vi "Custom Device CORE.vi"(8 "error in (no error)":errorcluster, 11 "CDW_MetaDataObj":refnum<class "NIVS_Consolidated_CDW_MetaDataObj.lvclass">) -> (0 "error out":errorcluster)   [LabVIEW 2020, in "NIVS_Consolidated_CDW_MetaDataObj.lvclass"]
doc: "This VI is the Core VI for the Custom Device Wizard.\n\nWritten by:\nStephan Daunke\n\nDate:\n2014/01/27\n\nCompany:\nNational Instruments Germany GmbH"
uses:
  NIVS_Consolidated_CDW_MetaDataObj.lvclass
  C:/Program Files/National Instruments/LabVIEW 2024/resource/dialog/NewProjectWizard/MetaDataObj/MetaDataObj.lvclass
  Action.ctl
  Internal data.ctl
  <resource>/dialog/NewProjectWizard/MetaDataObj/MetaDataObj.lvclass/MetaDataObj.ctl
  NIVS_Consolidated_CDW_MetaDataObj.lvclass/NIVS_Consolidated_CDW_MetaDataObj.ctl
  Template Classes/NIVS_CD Template/NIVS_CD Template.lvclass/NIVS_CD Template.ctl
  Template Classes/NIVS_PPLCD Template/NIVS_PPLCD Template.lvclass
  Utility folder.ctl
  CD Shared lvlib.ctl
  Common.ctl
  Add Item - Type.ctl
  CD System Explorer lvlib.ctl
  <vilib>/Utility/traverseref.llb/TRef TravTarget.ctl
  CD Engine lvlib.ctl
  Build Spec System Explorer.ctl
  Build Spec Engine.ctl
  <resource>/dialog/NewProjectWizard/MetaDataObj/Accessors/Read Project Root.vi
  Read CD Template.vi
  Template Classes/NIVS_CD Template/Read Extra Page Names.vi
  <resource>/dialog/NewProjectWizard/MetaDataObj/Accessors/Read Project Name.vi
  Template Classes/NIVS_CD Template/Read Support Runtime Configuration.vi
  Utility folder.vi
  CD Shared lvlib.vi
  Common.vi
  CD System Explorer lvlib.vi
  CD Engine lvlib.vi
  Build Spec System Explorer.vi
  Build Spec Engine.vi
  Template Classes/NIVS_CD Template/NIVS_CD Template.lvclass
  <vilib>/Utility/Data Type/NI_Data Type.lvlib
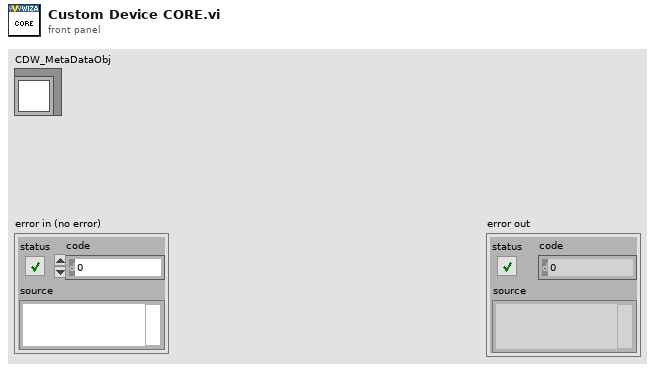
[diagram p1: front panel]
types:
  T1 = typedef "NIVS_Consolidated_CDW_MetaDataObj.lvclass/Internal data.ctl" = cluster{"CD GUID":string, "Extra Page GUIDs":string[], "System Explorer Library":refnum<vi>, "Shared Library":refnum<vi>, "Engine Library":refnum<vi>}
  T2 = typedef "NIVS_Consolidated_CDW_MetaDataObj.lvclass/Action.ctl" = enum16{"Project - Create Custom Device folder", "PC - Create GUID for each extra page", "PC-Utility - Create folder and copy -Copy .LLB to NI VeriStand dir-", "PC-Utility - Change -Copy .LLB to NI VeriStand dir-", "PC-Shared - Create folder and copy Constants.vi", "PC-Shared - Change Constants.vi content", "PC-Shared - Create library", "PC-Shared - Add folders and VIs to library", "PC-System Explorer - Create folder and copy templates", "PC-System Explorer - Create extra pages", "PC-System Explorer - Create library", "PC-System Explorer - Add folders and VIs to library", "PC-Engine - Create folder and copy the RT Template", "PC-Engine - Create library", "PC-Engine - Add virtual folders and VIs to library", "PC-XML - Create and change file", "PC-Help - Copy HTML Files", "Project - Read project file content", "Project - Edit Utility section", "Project - Edit XML section", "Project - Edit Engine Library section", "Project - Edit Shared Library section", "Project - Edit System Explorer Library section", "Project - Edit Custom Device Name", "Project - Edit System Explorer LLB Name", "Project - Edit Engine LLB OS dependent file name", "Project - Copy Configuration file", "Project - Write new project file"}
  T3 = typedef "NIVS_Consolidated_CDW_MetaDataObj.lvclass/Utility folder.ctl" = enum16{"Utility.FolderName", "Utility.PPL Tools Folder Path", "Utility.Copy .llb to NI VeriStand dir.FileName", "Utility.Copy .llb to NI VeriStand dir.FilePathAndName", "Utility.LLB Pre Build.FilePathAndName", "Utility.PPL Pre Build.FileName", "Utility.XMLUpdater.FileName", "Utility.XMLUpdater.FolderName", "Utility.XMLUpdater.Library.FileName"}
  T4 = typedef "NIVS_Consolidated_CDW_MetaDataObj.lvclass/CD Shared lvlib.ctl" = enum16{"LibraryFileName", "LibraryFolderName", "ConstantsVI.VIPathAndName", "Shared.FolderName", "Shared.Types.FolderName", "Shared.Constants.VIName", "Shared.Constants.VITemplateName", "Shared.Constants.VITemplatePathAndName", "Shared.CompiledSettings.RelativePath", "Shared.Constants.RelativePath", "Shared.CompiledSettings.Name", "Shared.CompiledSettings.Name.NoExtension", "Shared.CompiledSettings.ClusterName"}
  T5 = typedef "NIVS_Consolidated_CDW_MetaDataObj.lvclass/Common.ctl" = enum16{"ProjectName", "TemplatesFolderName", "PPLTemplatesFolderName", "ProjectTemplatePathAndName", "ProjectPPLTemplatePathAndName", "TimingAndSyncFolderName", "CustomDeviceFolderName", "PathToTemplates", "PathToPPLTemplates", "PathToExplorerPPLTemplates", "PathToEnginePPLTemplates", "PathToConfigurationFile", "ProjectConfigurationName"}
  T6 = typedef "NIVS_Consolidated_CDW_MetaDataObj.lvclass/Add Item - Type.ctl" = string
  T7 = typedef "NIVS_Consolidated_CDW_MetaDataObj.lvclass/CD System Explorer lvlib.ctl" = enum16{"LibraryFileName", "LibraryFolderName", "System Explorer.FolderName", "System Explorer.Dynamically Called.FolderName", "System Explorer.Dynamically Called.Extra Pages.FolderName", "System Explorer.Dynamically Called.Extra Pages.TemplatePathAndName", "System Explorer.Dynamically Called.Main Page.VIName", "System Explorer.Dynamically Called.Main Page.TemplatePathAndName", "System Explorer.Dynamically Called.Initialization VI.VIName", "System Explorer.Dynamically Called.Initialization VI.TemplatePathAndName", "System Explorer.SubVI.FolderName", "System Explorer.Types.FolderName", "System Explorer.ActionVIOnCompile.VIName", "System Explorer.ActionVIOnRecompile.VIName", "System Explorer.ExportConfigRTM.VIName", "System Explorer.PPL.ExportConfigRTM.VIName", "System Explorer.LoadHelpFile.VIName", "System Explorer.PPL.LoadHelpFile.VIName", "System Explorer.SetRTDriverVIsFilePaths.VIName", "System Explorer.ClearRTDriverVIs.VIName"}
  T8 = typedef "TRef TravTarget.ctl" = enum16{"FP", "BD", "Other"}
  T9 = typedef "NIVS_Consolidated_CDW_MetaDataObj.lvclass/CD Engine lvlib.ctl" = enum16{"LibraryFileName", "LibraryFolderName", "Engine.FolderName", "Engine.Init.FolderName", "Engine.Run.FolderName", "Engine.Shutdown.FolderName", "Types.FolderName", "Engine.RT Driver VI.TemplatePath", "Engine.RT Driver VI.FileName", "Engine.PPL.RT Driver VI_InlineAsync.FileName", "Engine.RTStateVariables.Name", "Engine.PPL.RTStateVariables.Name", "Engine.RTStateVariables.Name.NoExtension", "Engine.Async.NameExtension", "Engine.Async.TemplateName", "Engine.PPL.Async.TemplateName", "Engine.PPL.Async.InitVSGlobals.Name", "Engine.PPL.RT Driver VI_Inline.FileName"}
  T10 = typedef "NIVS_Consolidated_CDW_MetaDataObj.lvclass/Build Spec System Explorer.ctl" = enum16{"Destinations.LLBFileName", "Destinations.PPLFileName"}
  T11 = typedef "NIVS_Consolidated_CDW_MetaDataObj.lvclass/Build Spec Engine.ctl" = enum16{"Destinations.LLBWindowsFileName", "Destinations.LLBLinux64FileName", "Destinations.PPLWindowsFileName", "Destinations.PPLLinux64FileName"}
  T12 = enum16{"open", "replace", "create", "open or create", "replace or create", "replace or create with confirmation"}
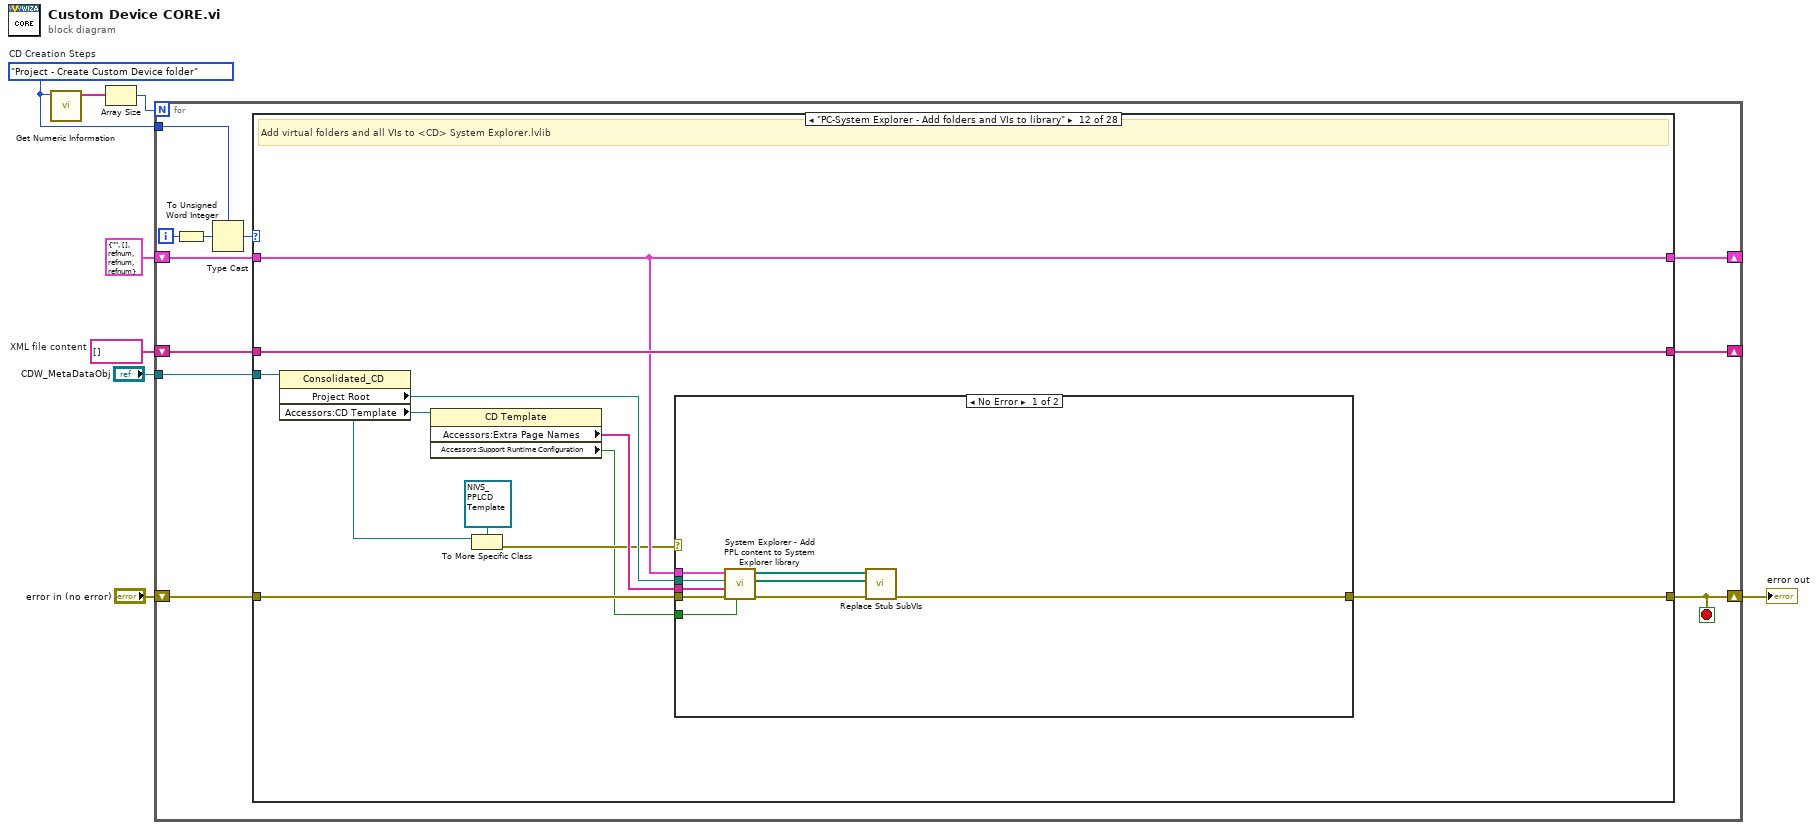
[diagram p0: block diagram]
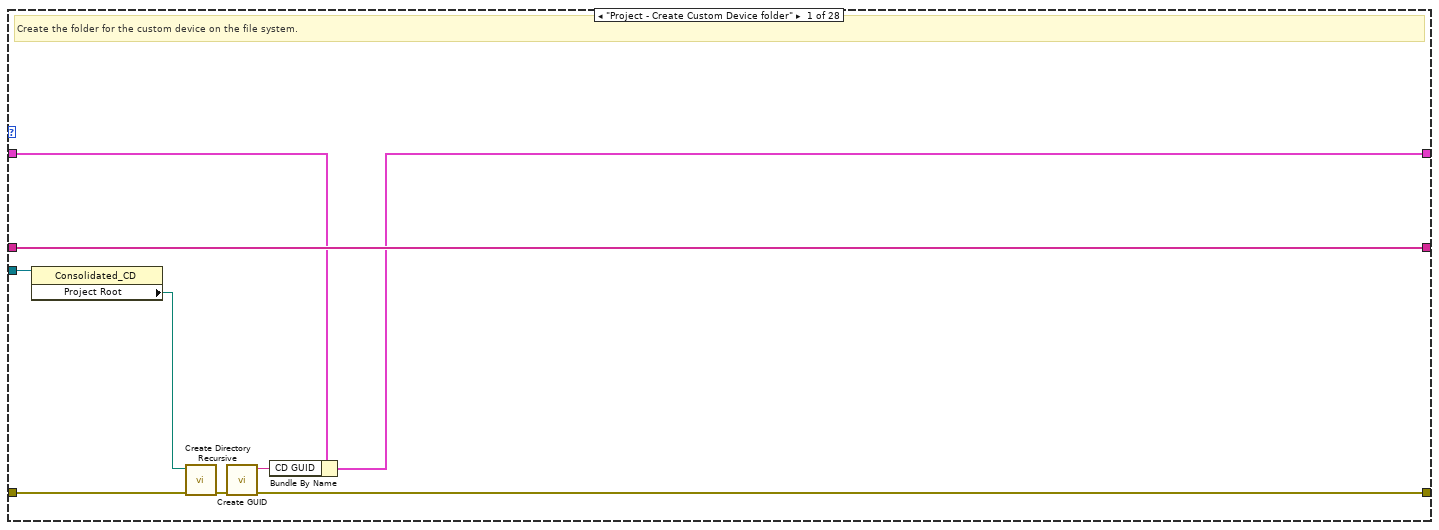
[diagram p2: hidden frame]
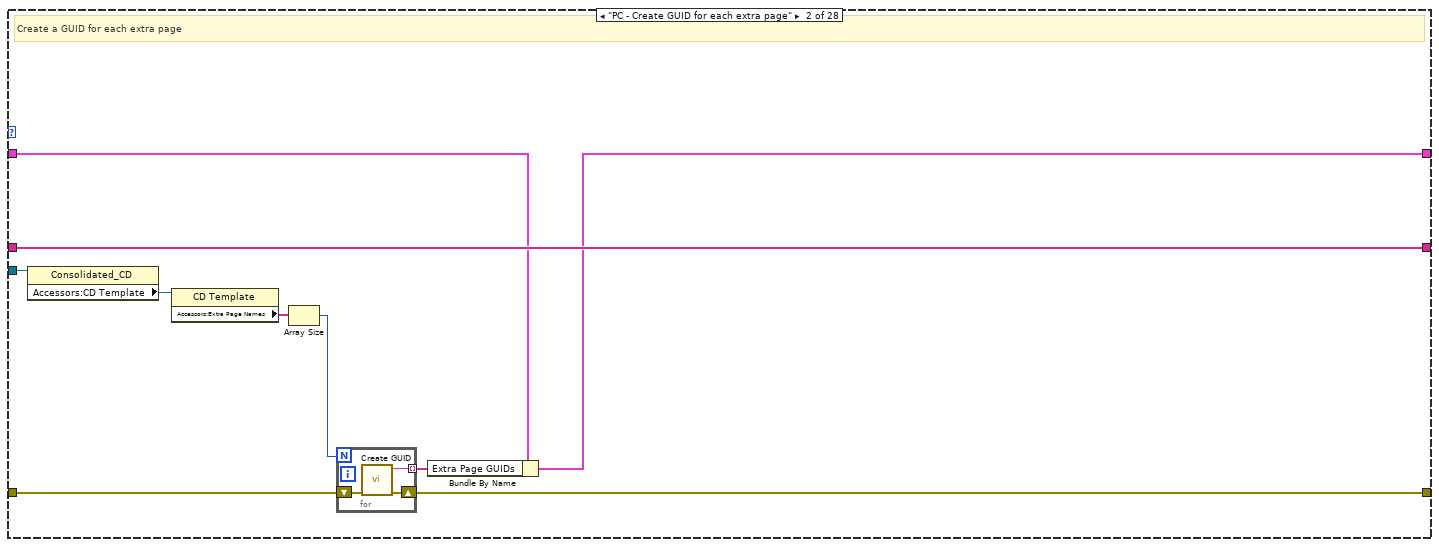
[diagram p3: hidden frame]
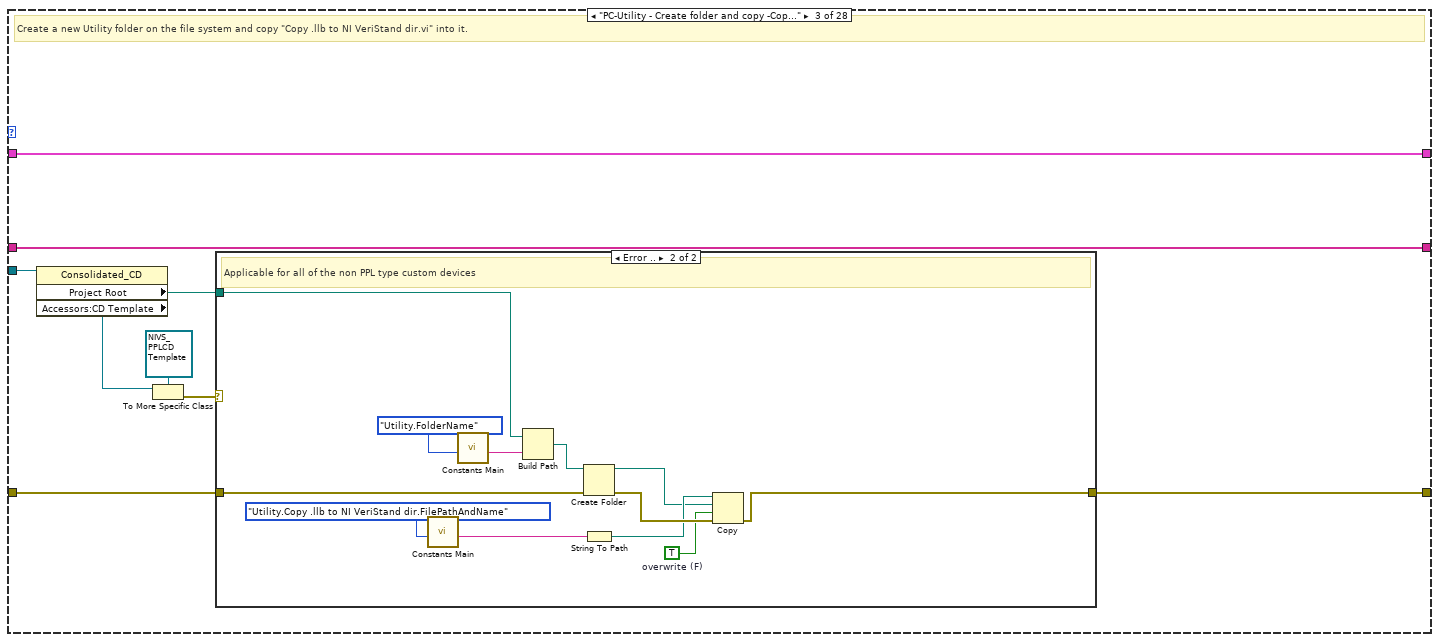
[diagram p4: hidden frame]
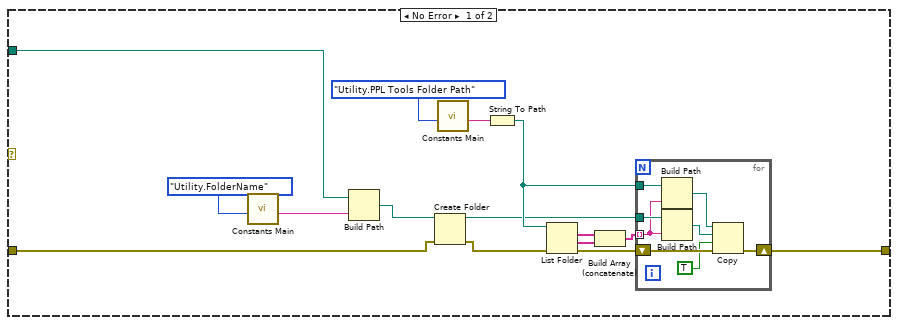
[diagram p5: hidden frame]
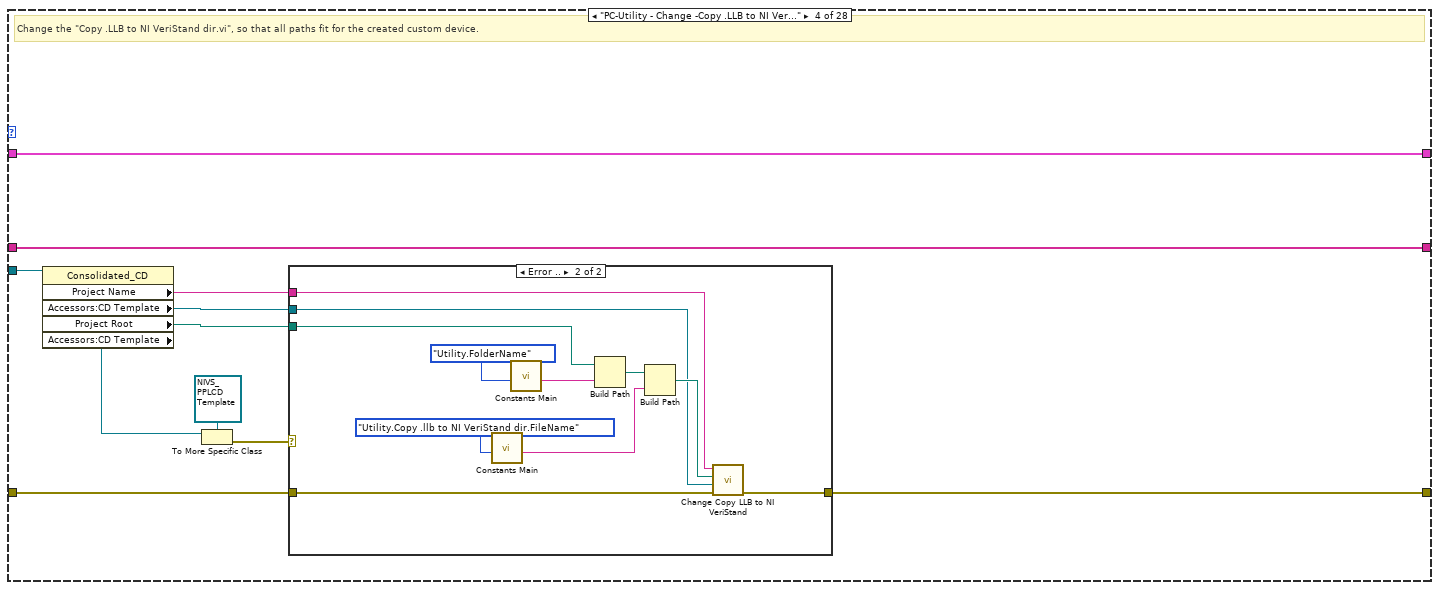
[diagram p6: hidden frame]
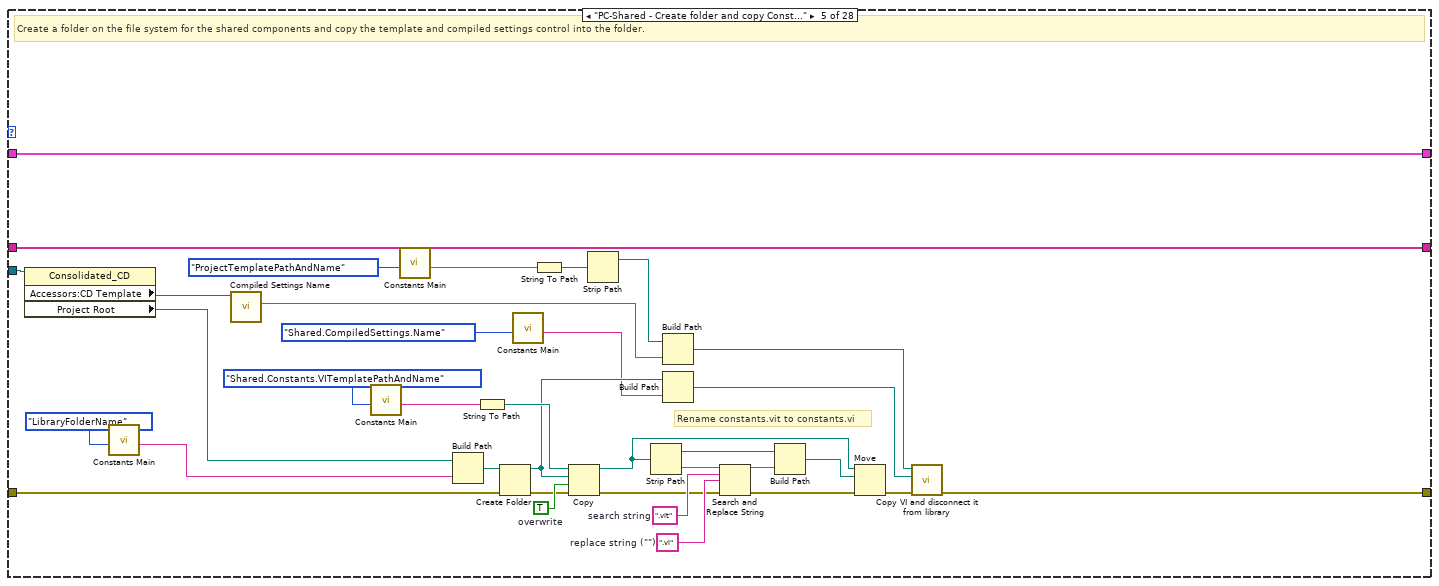
[diagram p8: hidden frame]
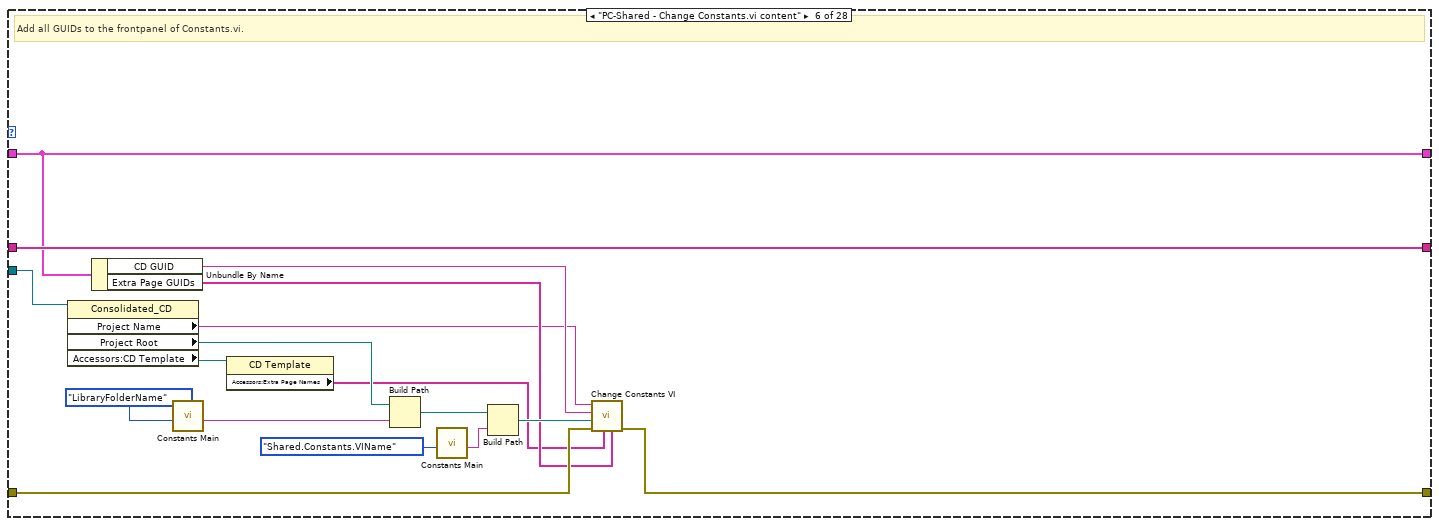
[diagram p9: hidden frame]
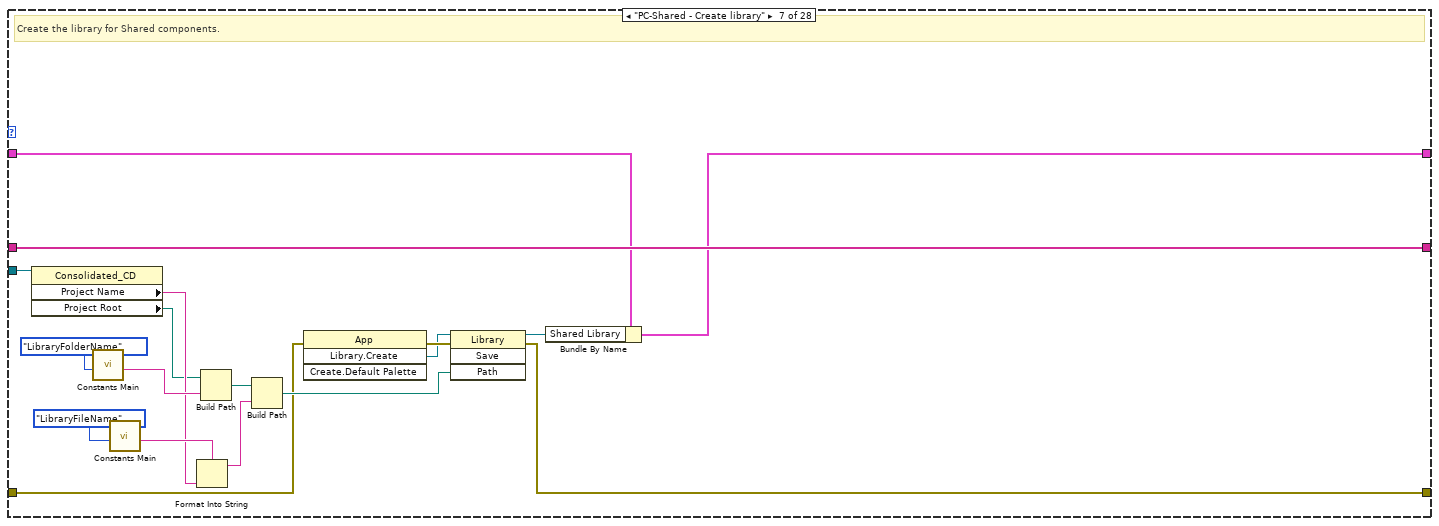
[diagram p10: hidden frame]
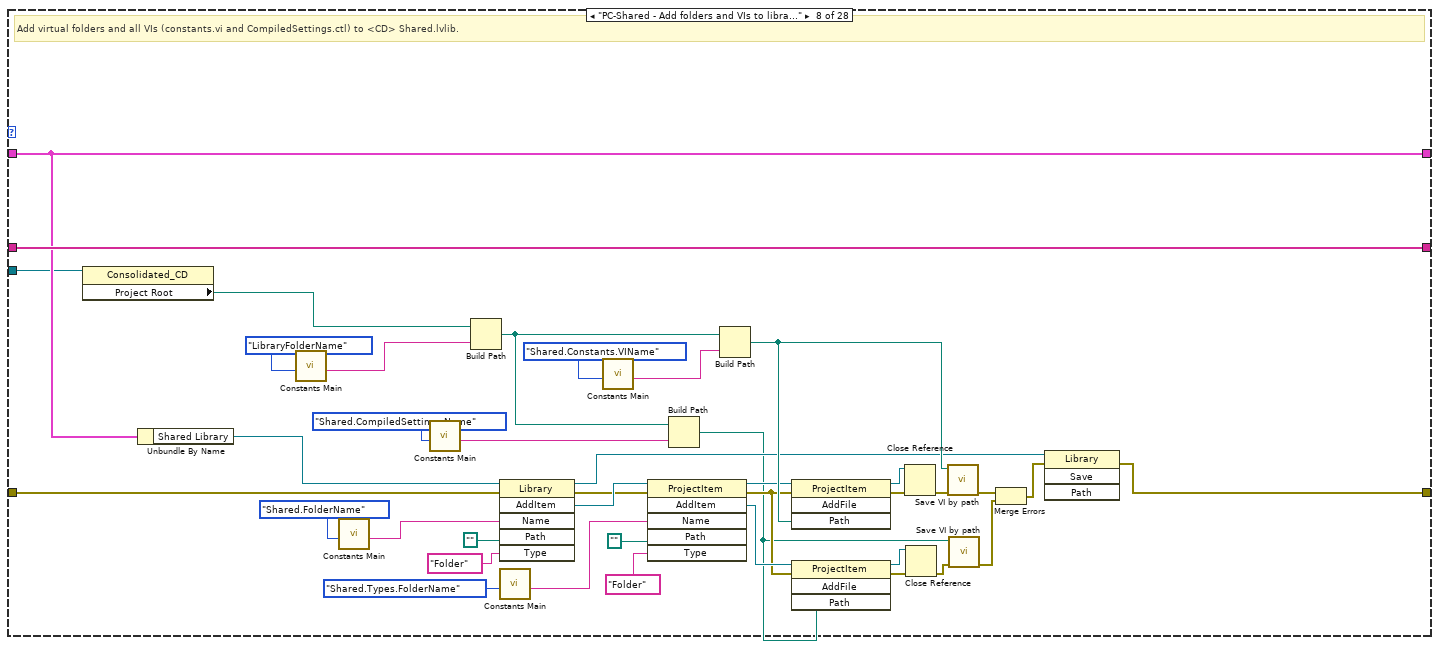
[diagram p11: hidden frame]
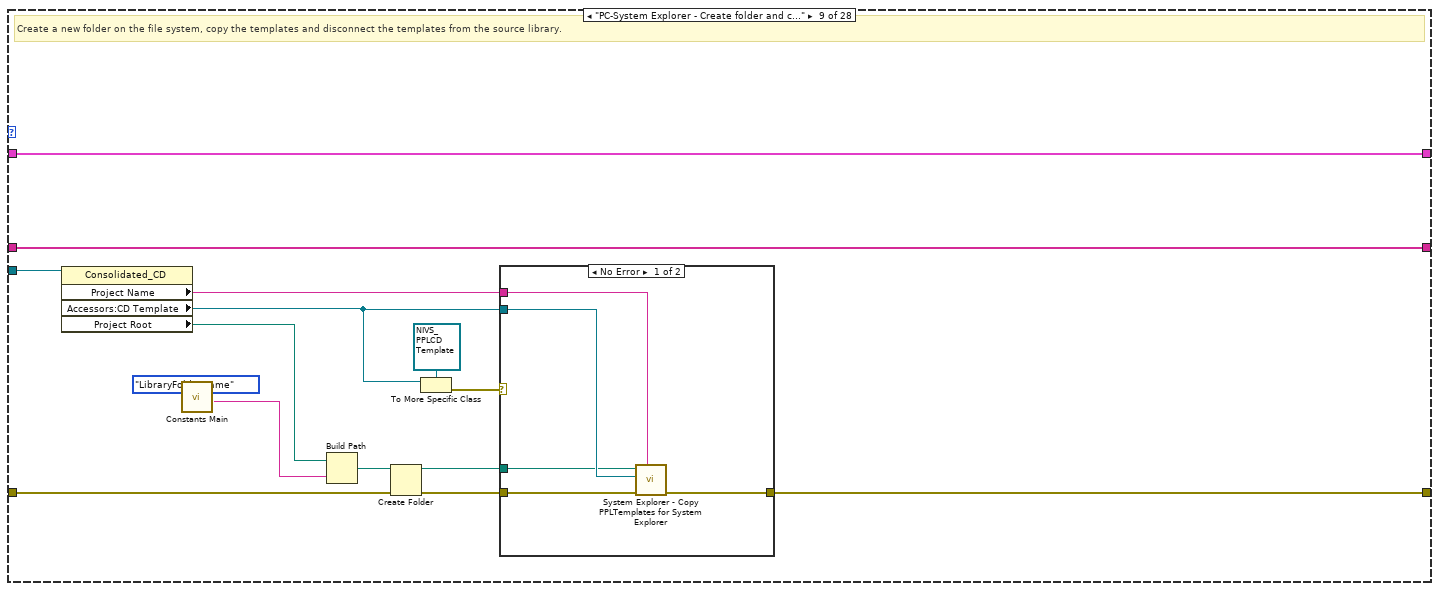
[diagram p12: hidden frame]
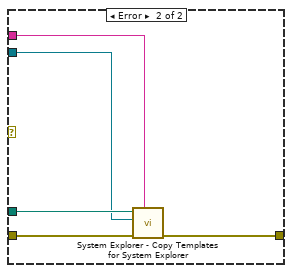
[diagram p13: hidden frame]
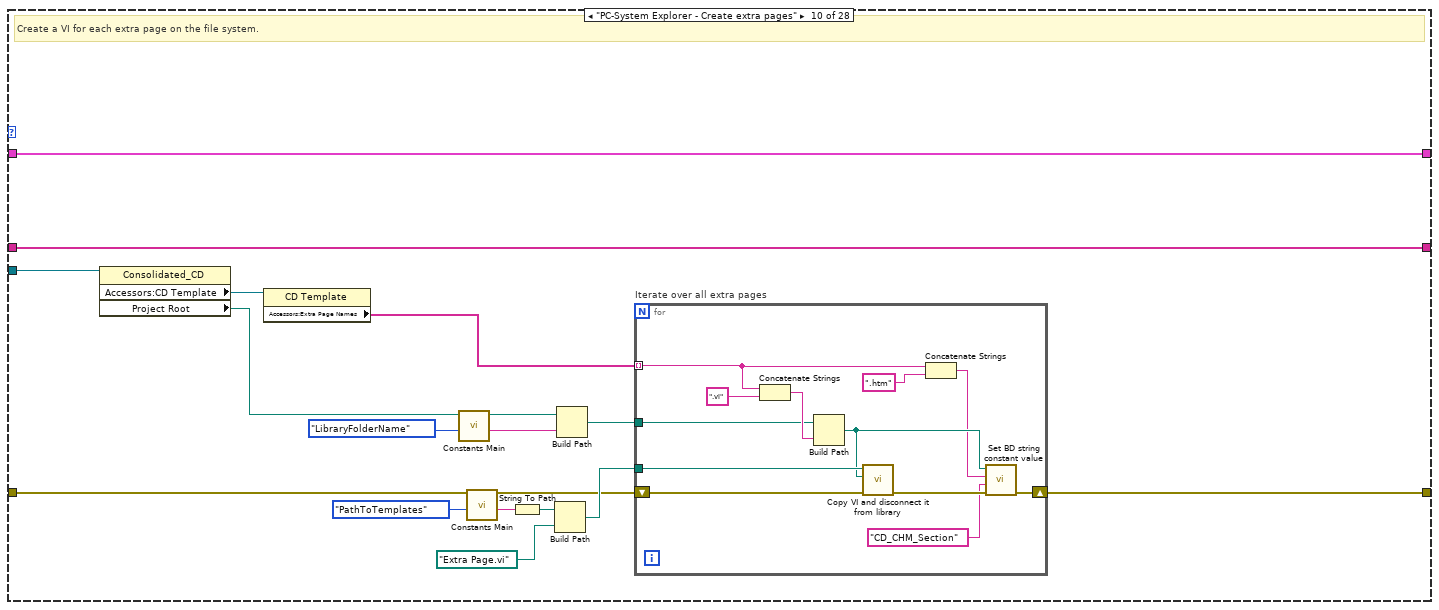
[diagram p14: hidden frame]
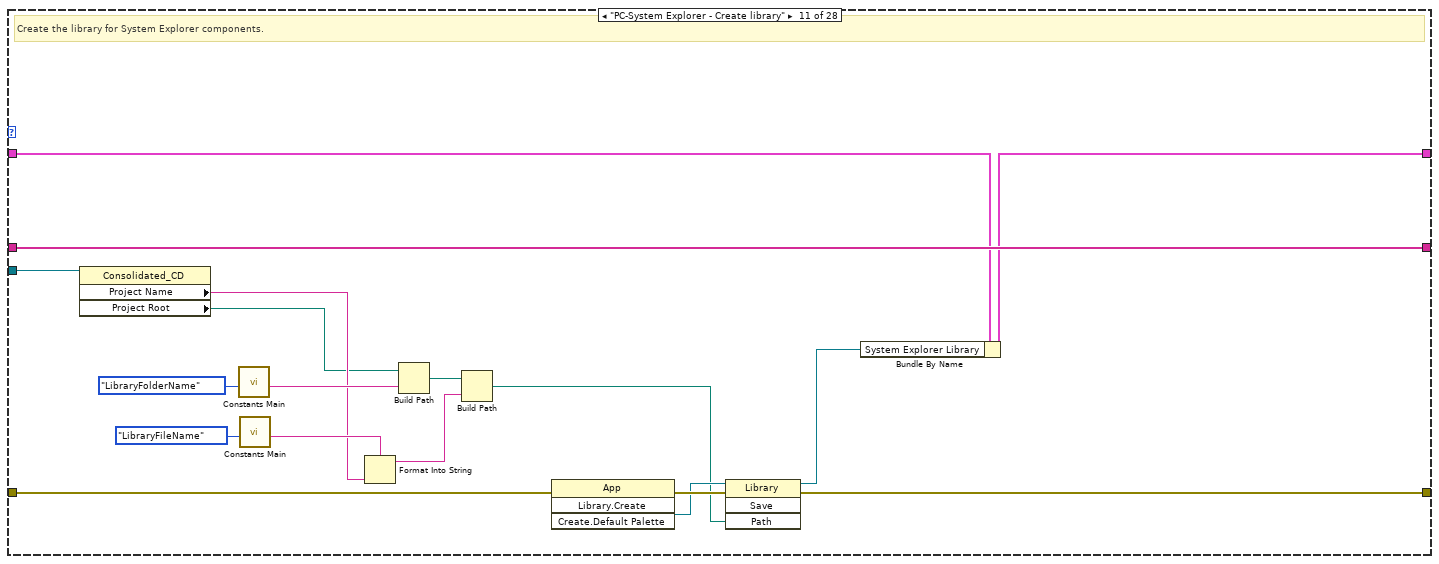
[diagram p15: hidden frame]
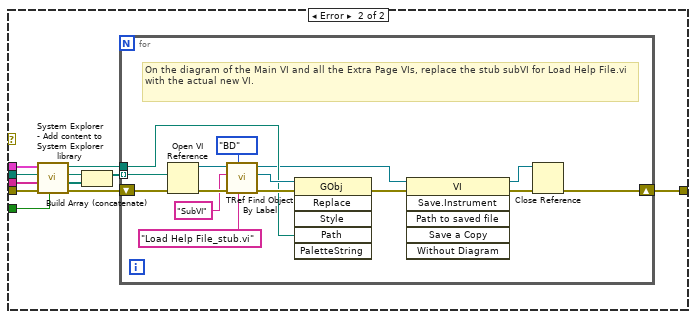
[diagram p16: hidden frame]
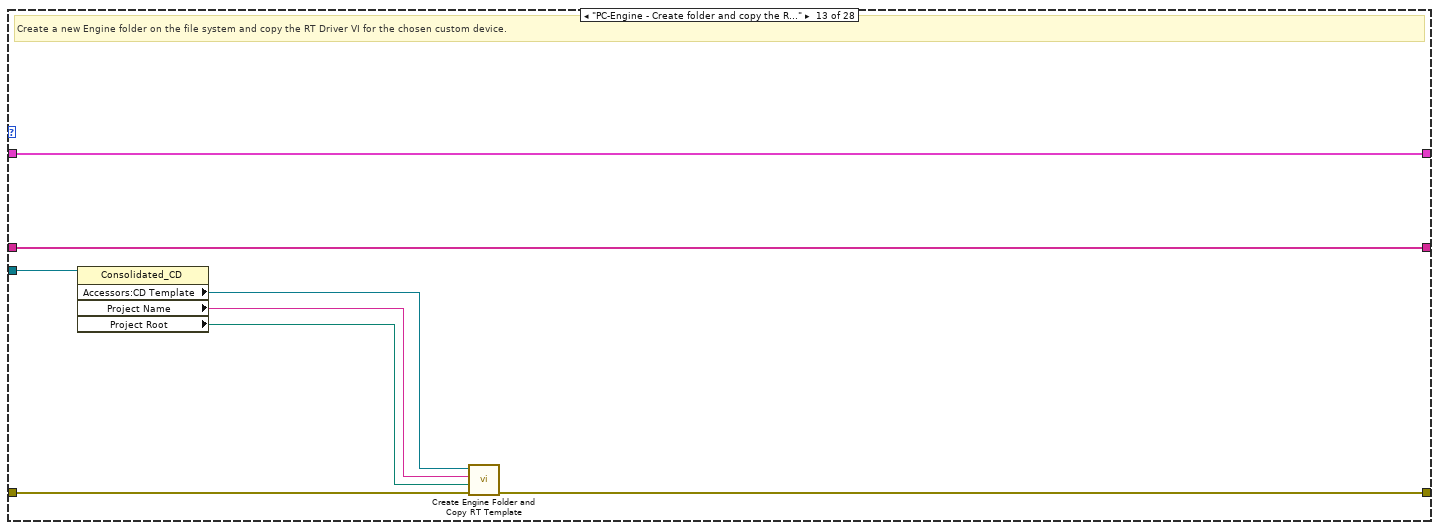
[diagram p17: hidden frame]
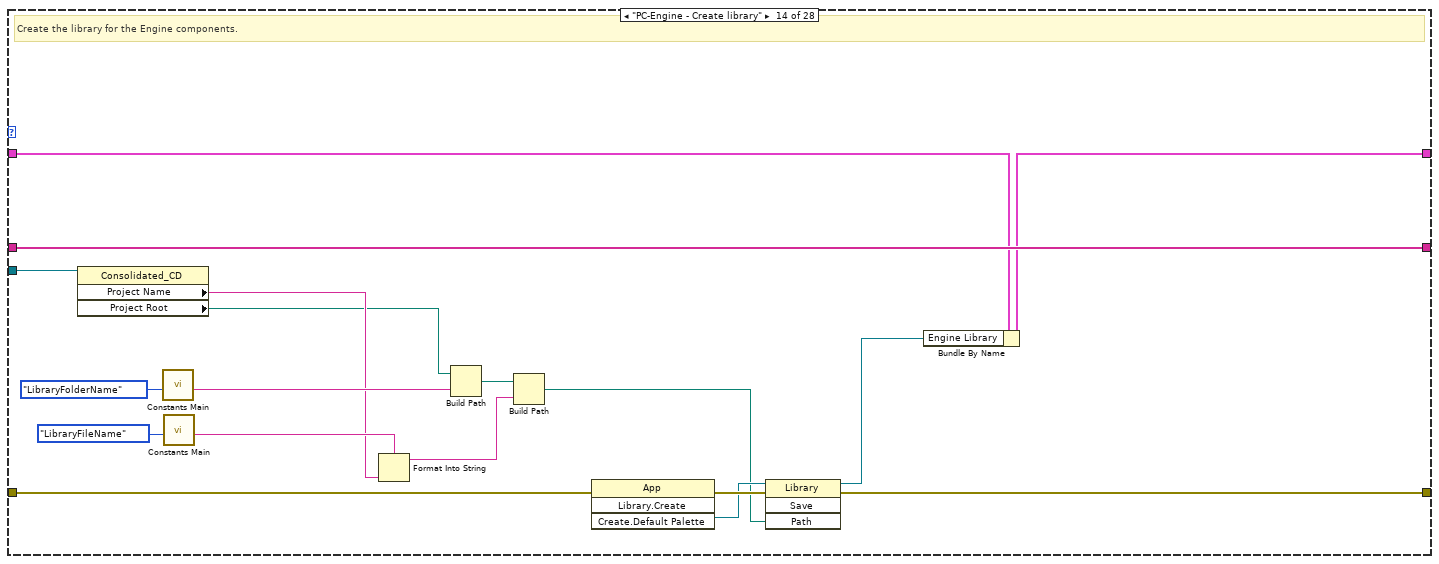
[diagram p18: hidden frame]
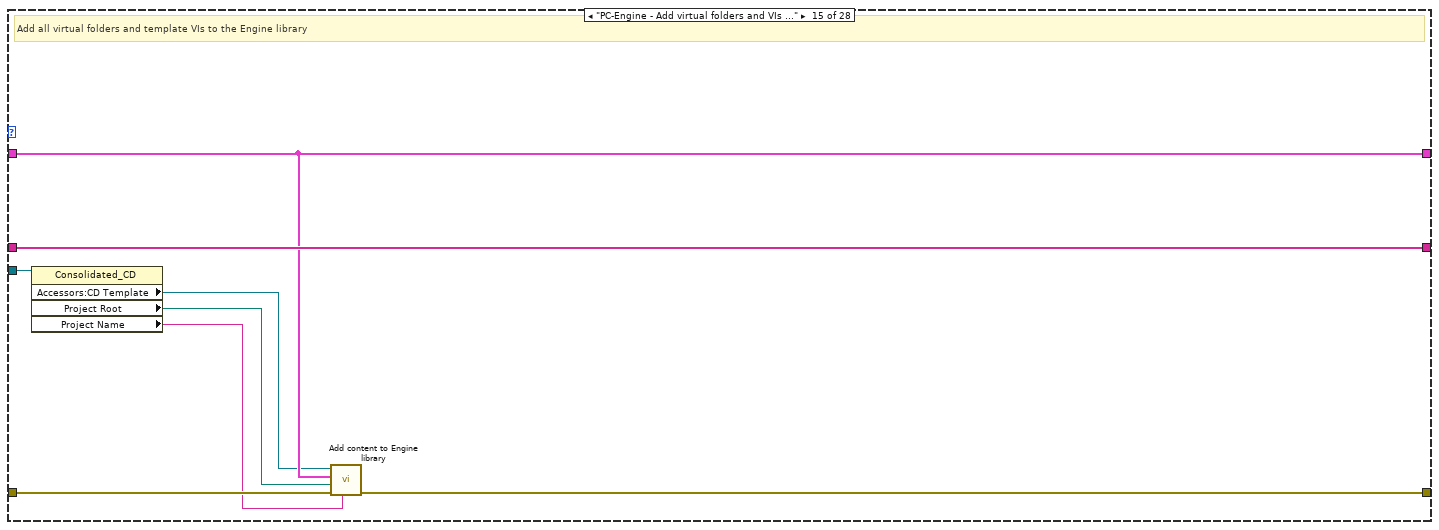
[diagram p19: hidden frame]
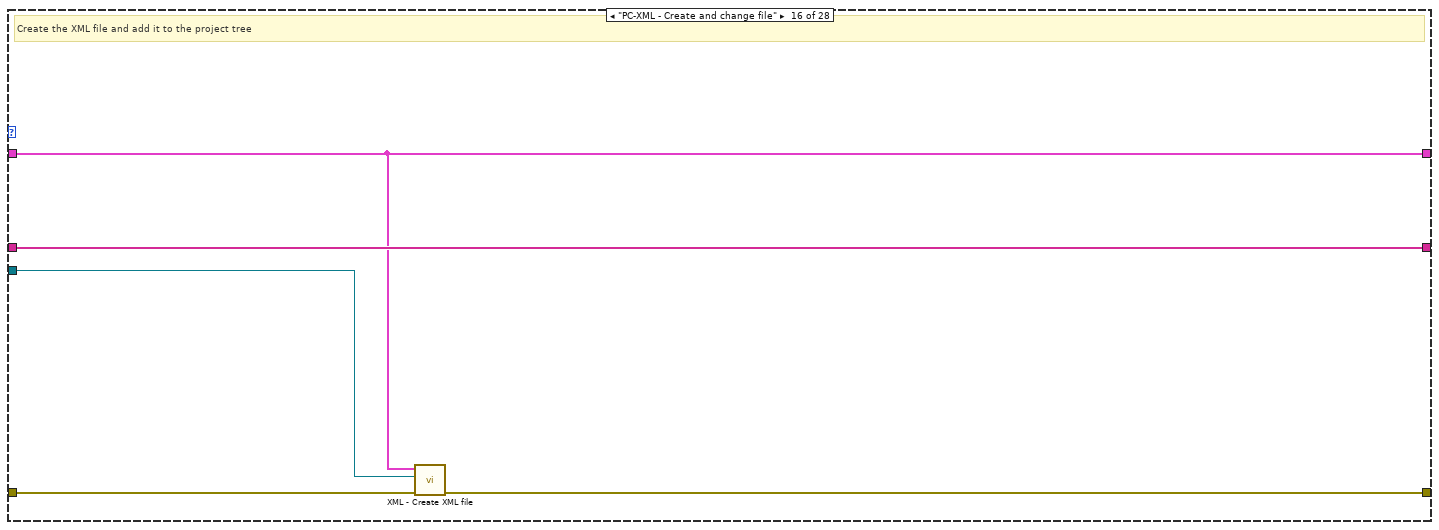
[diagram p20: hidden frame]
diagram:
  w4 = Action."Project - Create Custom Device folder"  # CD Creation Steps
  w5 = string[] []  # XML file content
  n1 = call <vilib>:"Get Numeric Information.vi"("variant"=w4) -> ("enum names"=w3:string[])  [unwired: 7 in, 3 out]
  n2 = Array Size(array=w3) -> (size(s)=w2:i32)
  n3 = for {
    N: w2 -> [_]
    shift-right: [w16] -> _
    shift-left: T1 {"CD GUID"="", "Extra Page GUIDs"=[], "System Explorer Library"=refnum, "Shared Library"=refnum, "Engine Library"=refnum} ("CD Wizard - Internal Data") -> [w18]
    shift-right: [w15] -> _
    shift-left: w5 -> [w17]
    shift-right: [w14] -> w6
    shift-left: "error in (no error)" -> [w19]
    tunnel: w4 -> [w12]
    tunnel: "CDW_MetaDataObj" -> [w11]
    i -> [w13]
    stop <- w14 stop-if-true
    n4 = To Unsigned Word Integer(number=w13) -> (unsigned 16bit integer=w10:u16)
    n5 = Type Cast(type=w12, x=w10) -> (*(type *) &x=w9:T2)
    n6 = case shown="\"PC-System Explorer - Add folders and VIs to library\"" w9 {
      tunnel: w19 -> [w24 w37 w46 w91 w113 w153 w164 w181 w223 w247 w274 w298 w341 w346 w367 w372 w387 w406 w428 w485 w504 w508 w539 w572 w586 w629 w687 w705]
      tunnel: [w25 w36 w49 w95 w115 w159 w165 w179 w218 w257 w275 w290 w335 w349 w361 w369 w378 w400 w421 w490 w503 w518 w542 w571 w590 w630 w686 w712] -> w14
      tunnel: w18 -> [w22 w34 w48 w94 w114 w150 w168 w199 w226 w256 w280 w297 w340 w353 w365 w371 w383 w416 w429 w487 w502 w509 w540 w568 w589 w632 w699 w736]
      tunnel: w17 -> [w28 w38 w50 w96 w143 w160 w178 w217 w232 w258 w288 w299 w342 w360 w368 w373 w392 _ w424 w489 w501 w513 w541 w569 w588 w631 w698 w730]
      tunnel: [w27 w33 w48 w94 w114 w150 w167 w199 w226 w256 w281 w297 w340 w352 w365 w371 w383 w416 w429 w487 w502 w509 w540 w568 w589 w632 w699 w736] -> w16
      tunnel: [w28 w38 w50 w96 w143 w160 w178 w217 w232 w258 w288 w299 w342 w360 w368 w373 w392 w410 w422 w488 w505 w519 w536 w570 w587 w627 w698 w730] -> w15
      tunnel: w11 -> [w21 w32 w45 w93 w112 w152 w163 w183 w225 w246 w273 w296 w339 w345 w366 w370 w377 w405 w425 w484 w500 w507 w538 w567 w583 w625 w692 w704]
      frame "Project - Create Custom Device folder" {
        # "Create the folder for the custom device on the file system."
        n7 = property class="Consolidated_CD"(reference=w21) -> ("Project Root"=w20:path)  [unwired: 1 in, 2 out]
        n8 = call <vilib>:"Create Directory Recursive.vi"("error in (no error)"=w24, "directory"=w20) -> ("error out"=w23:errorcluster)  [unwired: 3 in, 2 out]
        n9 = call "Create GUID.vi"("error in (no error)"=w23) -> ("error out"=w25:errorcluster, "Generated GUID"=w26:string)  [unwired: 9 in]
        n10 = Bundle By Name(cluster=w22, "CD GUID"=w26) -> (w27:T1)
      }
      frame "PC - Create GUID for each extra page" {
        # "Create a GUID for each extra page"
        n11 = property class="Consolidated_CD"(reference=w32) -> ("Accessors:CD Template"=w31:refnum<class "NIVS_CD Template.lvclass">)  [unwired: 1 in, 2 out]
        n12 = property class="CD Template"(reference=w31) -> ("Accessors:Extra Page Names"=w30:string[])  [unwired: 1 in, 2 out]
        n13 = Array Size(array=w30) -> (size(s)=w29:i32)
        n14 = for {
          N: w29 -> [_]
          shift-right: [w40] -> w36
          shift-left: w37 -> [w41]
          tunnel: [w39] -> w35 mode=indexing
          n15 = call "Create GUID.vi"("error in (no error)"=w41) -> ("error out"=w40:errorcluster, "Generated GUID"=w39:string)  [unwired: 9 in]
        }
        n16 = Bundle By Name(cluster=w34, "Extra Page GUIDs"=w35) -> (w33:T1)
      }
      frame "PC-Utility - Create folder and copy -Copy .LLB to NI VeriStand dir-" {
        # "Create a new Utility folder on the file system and copy \"Copy .llb to NI VeriStand dir.vi\" into it."
        n17 = property class="Consolidated_CD"(reference=w45) -> ("Project Root"=w47:path, "Accessors:CD Template"=w42:refnum<class "NIVS_CD Template.lvclass">)  [unwired: 1 in, 2 out]
        n18 = To More Specific Class(target class=refnum<class "NIVS_PPLCD Template.lvclass"> refnum ("NIVS_PPLCD Template.lvclass"), reference=w42) -> (error out=w43:errorcluster)  [unwired: 1 in, 1 out]
        n19 = case shown="Error .." w43 {
          tunnel: [w51 w74] -> w49
          tunnel: w47 -> [w59 w76]
          tunnel: w46 -> [w60 w75]
          frame No Error {
            n20 = call-poly "Constants Main.vi"("Action"=Utility_folder."Utility.FolderName") -> ("Output"=w61:string)  [unwired: 10 in]
            n21 = Build Path(base path=w59, name or relative path=w61) -> (appended path=w65:path)
            n22 = Create Folder(path (use dialog)=w65, error in=w60) -> (created path=w56:path, error out=w55:errorcluster)  [unwired: 1 in, 1 out]
            n23 = call-poly "Constants Main.vi"("Action"=Utility_folder."Utility.PPL Tools Folder Path") -> ("Output"=w63:string)  [unwired: 10 in]
            n24 = String To Path(string=w63) -> (path=w57:path)
            n25 = List Folder(path=w57, error in=w55) -> (filenames=w54:string[], folder names=w53:string[], error out=w58:errorcluster)  [unwired: 2 in, 1 out]
            n26 = Build Array (concatenate)(w54, w53) -> (w52:string[])
            n27 = for {
              tunnel: w52 -> [w68] mode=indexing
              tunnel: w57 -> [w71]
              shift-right: [w72] -> w51
              shift-left: w58 -> [w73]
              tunnel: w56 -> [w69]
              n28 = Build Path(base path=w71, name or relative path=w68) -> (appended path=w70:path)
              n29 = Build Path(base path=w69, name or relative path=w68) -> (appended path=w67:path)
              n30 = Copy(8:w73, 9:TRUE ("overwrite (F)"), 10:w67, 11:w70) -> (0:w72:errorcluster)  [unwired: 1 in, 2 out]
            }
          }
          frame Error {
            w83 = TRUE  # overwrite (F)
            # "Applicable for all of the non PPL type custom devices"
            n31 = call-poly "Constants Main.vi"("Action"=Utility_folder."Utility.Copy .llb to NI VeriStand dir.FilePathAndName") -> ("Output"=w81:string)  [unwired: 10 in]
            n32 = call-poly "Constants Main.vi"("Action"=Utility_folder."Utility.FolderName") -> ("Output"=w78:string)  [unwired: 10 in]
            n33 = Build Path(base path=w76, name or relative path=w78) -> (appended path=w85:path)
            n34 = Create Folder(path (use dialog)=w85, error in=w75) -> (created path=w77:path, error out=w84:errorcluster)  [unwired: 1 in, 1 out]
            n35 = String To Path(string=w81) -> (path=w80:path)
            n36 = Copy(8:w84, 9:w83, 10:w77, 11:w80) -> (0:w74:errorcluster)  [unwired: 3 out]
          }
        }
      }
      frame "PC-Utility - Change -Copy .LLB to NI VeriStand dir-" {
        # "Change the \"Copy .LLB to NI VeriStand dir.vi\", so that all paths fit for the created custom device."
        n37 = property class="Consolidated_CD"(reference=w93) -> ("Project Name"=w92:string, "Accessors:CD Template"=w88:refnum<class "NIVS_CD Template.lvclass">, "Project Root"=w90:path, "Accessors:CD Template"=w87:refnum<class "NIVS_CD Template.lvclass">)  [unwired: 1 in, 2 out]
        n38 = To More Specific Class(target class=refnum<class "NIVS_PPLCD Template.lvclass"> refnum ("NIVS_PPLCD Template.lvclass"), reference=w87) -> (error out=w86:errorcluster)  [unwired: 1 in, 1 out]
        n39 = case shown="Error .." w86 {
          tunnel: [w97 w103] -> w95
          tunnel: w92 -> [_ w101]
          tunnel: w91 -> [w97 w100]
          tunnel: w90 -> [_ w99]
          tunnel: w88 -> [_ w98]
          frame No Error {
            # "No need to do this for the PPL based CDs"
          }
          frame Error {
            n40 = call-poly "Constants Main.vi"("Action"=Utility_folder."Utility.Copy .llb to NI VeriStand dir.FileName") -> ("Output"=w104:string)  [unwired: 10 in]
            n41 = call-poly "Constants Main.vi"("Action"=Utility_folder."Utility.FolderName") -> ("Output"=w106:string)  [unwired: 10 in]
            n42 = Build Path(base path=w99, name or relative path=w106) -> (appended path=w105:path)
            n43 = Build Path(base path=w105, name or relative path=w104) -> (appended path=w102:path)
            n44 = call "Change Copy LLB to NI VeriStand.vi"("error in (no error)"=w100, "CD Template"=w98, "Copy .LLB to ... path"=w102, "CD Name"=w101) -> ("error out"=w103:errorcluster)  [unwired: 7 in]
          }
        }
      }
      frame "PC-Shared - Create folder and copy Constants.vi" {
        w132 = ".vi"  # replace string ("")
        w133 = ".vit"  # search string
        w137 = TRUE  # overwrite
        # "Rename constants.vit to constants.vi"
        # "Create a folder on the file system for the shared components and copy the template and compiled settings control into the folder."
        n45 = property class="Consolidated_CD"(reference=w112) -> ("Accessors:CD Template"=w110:refnum<class "NIVS_CD Template.lvclass">, "Project Root"=w111:path)  [unwired: 1 in, 2 out]
        n46 = call-poly "Constants Main.vi"("Action"=CD_Shared_lvlib."LibraryFolderName") -> ("Output"=w140:string)  [unwired: 10 in]
        n47 = call-dynamic "Compiled Settings Name.vi"("CD Template in"=w110) -> ("Compiled Settings Name"=w109:string)  [unwired: 10 in]
        n48 = call-poly "Constants Main.vi"("Action"=CD_Shared_lvlib."Shared.Constants.VITemplatePathAndName") -> ("Output"=w138:string)  [unwired: 10 in]
        n49 = call-poly "Constants Main.vi"("Action"=Common."ProjectTemplatePathAndName") -> ("Output"=w124:string)  [unwired: 10 in]
        n50 = Build Path(base path=w111, name or relative path=w140) -> (appended path=w142:path)
        n51 = String To Path(string=w138) -> (path=w130:path)
        n52 = Create Folder(path (use dialog)=w142, error in=w113) -> (created path=w121:path, error out=w131:errorcluster)  [unwired: 1 in, 1 out]
        n53 = call-poly "Constants Main.vi"("Action"=CD_Shared_lvlib."Shared.CompiledSettings.Name") -> ("Output"=w116:string)  [unwired: 10 in]
        n54 = String To Path(string=w124) -> (path=w123:path)
        n55 = Copy(8:w131, 9:w137, 10:w121, 11:w130) -> (0:w129:errorcluster, 3:w126:path)  [unwired: 2 out]
        n56 = Strip Path(path=w123) -> (stripped path=w122:path)  [unwired: 1 out]
        n57 = Strip Path(path=w126) -> (stripped path=w136:path, name=w135:string)
        n58 = Build Path(base path=w122, name or relative path=w109) -> (appended path=w120:path)
        n59 = Build Path(base path=w121, name or relative path=w116) -> (appended path=w119:path)
        n60 = Search and Replace String(input string=w135, search string=w133, replace string=w132, error in=w129) -> (result string=w134:string, error out=w128:errorcluster)  [unwired: 4 in, 2 out]
        n61 = Build Path(base path=w136, name or relative path=w134) -> (appended path=w127:path)
        n62 = Move(source path=w126, error in=w128, 10:w127) -> (error out=w118:errorcluster)  [unwired: 2 in, 2 out]
        n63 = call "Copy VI and disconnect it from library.vi"("error in (no error)"=w118, "VI Target Path"=w119, "VI Source Path"=w120) -> ("error out"=w115:errorcluster)  [unwired: 8 in]
      }
      frame "PC-Shared - Change Constants.vi content" {
        # "Add all GUIDs to the frontpanel of Constants.vi."
        n64 = property class="Consolidated_CD"(reference=w152) -> ("Project Name"=w146:string, "Project Root"=w151:path, "Accessors:CD Template"=w145:refnum<class "NIVS_CD Template.lvclass">)  [unwired: 1 in, 2 out]
        n65 = Unbundle By Name(w150) -> ("CD GUID"=w148:string, "Extra Page GUIDs"=w147:string[])
        n66 = call-poly "Constants Main.vi"("Action"=CD_Shared_lvlib."LibraryFolderName") -> ("Output"=w154:string)  [unwired: 10 in]
        n67 = property class="CD Template"(reference=w145) -> ("Accessors:Extra Page Names"=w144:string[])  [unwired: 1 in, 2 out]
        n68 = Build Path(base path=w151, name or relative path=w154) -> (appended path=w158:path)
        n69 = call-poly "Constants Main.vi"("Action"=CD_Shared_lvlib."Shared.Constants.VIName") -> ("Output"=w156:string)  [unwired: 10 in]
        n70 = Build Path(base path=w158, name or relative path=w156) -> (appended path=w149:path)
        n71 = call "Change Constants VI.vi"("Extra Page GUIDs"=w147, "Extra Page Names"=w144, "error in (no error)"=w153, "Constants.vi path"=w149, "CD GUID"=w148, "CD Name"=w146) -> ("error out"=w159:errorcluster)  [unwired: 5 in]
      }
      frame "PC-Shared - Create library" {
        # "Create the library for Shared components."
        n72 = property class="Consolidated_CD"(reference=w163) -> ("Project Name"=w162:string, "Project Root"=w161:path)  [unwired: 1 in, 2 out]
        n73 = call-poly "Constants Main.vi"("Action"=CD_Shared_lvlib."LibraryFolderName") -> ("Output"=w172:string)  [unwired: 10 in]
        n74 = call-poly "Constants Main.vi"("Action"=CD_Shared_lvlib."LibraryFileName") -> ("Output"=w173:string)  [unwired: 10 in]
        n75 = Format Into String(format string=w173, w162) -> (resulting string=w176:string)  [unwired: 2 in, 1 out]
        n76 = Build Path(base path=w161, name or relative path=w172) -> (appended path=w177:path)
        n77 = Build Path(base path=w177, name or relative path=w176) -> (appended path=w169:path)
        n78 = invoke class="App" method="Library.Create"(error in=w164) -> (error out=w171:errorcluster, "Create Library"=w170:refnum<vi>)  [unwired: 3 in, 2 out]
        n79 = invoke class="Library" method="Save"(reference=w170, error in=w171, "Path"=w169) -> (reference out=w166:refnum<vi>, error out=w165:errorcluster)  [unwired: 1 in, 2 out]
        n80 = Bundle By Name(cluster=w168, "Shared Library"=w166) -> (w167:T1)
      }
      frame "PC-Shared - Add folders and VIs to library" {
        # "Add virtual folders and all VIs (constants.vi and CompiledSettings.ctl) to <CD> Shared.lvlib."
        n81 = property class="Consolidated_CD"(reference=w183) -> ("Project Root"=w182:path)  [unwired: 1 in, 2 out]
        n82 = Unbundle By Name(w199) -> ("Shared Library"=w201:refnum<vi>)
        n83 = call-poly "Constants Main.vi"("Action"=CD_Shared_lvlib."LibraryFolderName") -> ("Output"=w196:string)  [unwired: 10 in]
        n84 = call-poly "Constants Main.vi"("Action"=CD_Shared_lvlib."Shared.FolderName") -> ("Output"=w197:string)  [unwired: 10 in]
        n85 = call-poly "Constants Main.vi"("Action"=CD_Shared_lvlib."Shared.CompiledSettings.Name") -> ("Output"=w188:string)  [unwired: 10 in]
        n86 = Build Path(base path=w182, name or relative path=w196) -> (appended path=w193:path)
        n87 = invoke class="Library" method="AddItem"(reference=w201, error in=w181, "Name"=w197, "Path"=path "", "Type"=T6 "Folder" ("Add Item - Type")) -> (reference out=w207:refnum<vi>, error out=w202:errorcluster, "AddItem"=w204:refnum<vi>)  [unwired: 1 in, 3 out]
        n88 = call-poly "Constants Main.vi"("Action"=CD_Shared_lvlib."Shared.Types.FolderName") -> ("Output"=w215:string)  [unwired: 10 in]
        n89 = call-poly "Constants Main.vi"("Action"=CD_Shared_lvlib."Shared.Constants.VIName") -> ("Output"=w184:string)  [unwired: 10 in]
        n90 = invoke class="ProjectItem" method="AddItem"(reference=w204, error in=w202, "Name"=w215, "Path"=path "", "Type"=T6 "Folder" ("Add Item - Type")) -> (reference out=w206:refnum<vi>, error out=w194:errorcluster, "AddItem"=w195:refnum<vi>)  [unwired: 1 in, 3 out]
        n91 = Build Path(base path=w193, name or relative path=w188) -> (appended path=w192:path)
        n92 = Build Path(base path=w193, name or relative path=w184) -> (appended path=w208:path)
        n93 = invoke class="ProjectItem" method="AddFile"(reference=w206, error in=w194, "Path"=w208) -> (reference out=w211:refnum<vi>, error out=w210:errorcluster)  [unwired: 1 in, 2 out]
        n94 = invoke class="ProjectItem" method="AddFile"(reference=w195, error in=w194, "Path"=w192) -> (reference out=w186:refnum<vi>, error out=w185:errorcluster)  [unwired: 1 in, 2 out]
        n95 = Close Reference(reference=w211, error in (no error)=w210) -> (error out=w212:errorcluster)
        n96 = Close Reference(reference=w186, error in (no error)=w185) -> (error out=w187:errorcluster)
        n97 = call "Save VI by path.vi"("error in (no error)"=w212, "VI path"=w208) -> ("error out"=w209:errorcluster)  [unwired: 9 in]
        n98 = call "Save VI by path.vi"("error in (no error)"=w187, "VI path"=w192) -> ("error out"=w190:errorcluster)  [unwired: 9 in]
        n99 = Merge Errors(w209, w190) -> (w191:errorcluster)
        n100 = invoke class="Library" method="Save"(reference=w207, error in=w191) -> (error out=w179:errorcluster)  [unwired: 2 in, 3 out]
      }
      frame "PC-System Explorer - Create folder and copy templates" {
        # "Create a new folder on the file system, copy the templates and disconnect the templates from the source library."
        n101 = property class="Consolidated_CD"(reference=w225) -> ("Project Name"=w224:string, "Accessors:CD Template"=w221:refnum<class "NIVS_CD Template.lvclass">, "Project Root"=w222:path)  [unwired: 1 in, 2 out]
        n102 = call-poly "Constants Main.vi"("Action"=CD_System_Explorer_lvlib."LibraryFolderName") -> ("Output"=w229:string)  [unwired: 10 in]
        n103 = Build Path(base path=w222, name or relative path=w229) -> (appended path=w231:path)
        n104 = Create Folder(path (use dialog)=w231, error in=w223) -> (created path=w227:path, error out=w228:errorcluster)  [unwired: 1 in, 1 out]
        n105 = To More Specific Class(target class=refnum<class "NIVS_PPLCD Template.lvclass"> refnum ("NIVS_PPLCD Template.lvclass"), reference=w221) -> (error out=w219:errorcluster)  [unwired: 1 in, 1 out]
        n106 = case shown="No Error" w219 {
          tunnel: w228 -> [w237 w242]
          tunnel: w227 -> [w233 w241]
          tunnel: [w236 w240] -> w218
          tunnel: w224 -> [w235 w239]
          tunnel: w221 -> [w234 w238]
          frame No Error {
            n107 = call "System Explorer - Copy PPLTemplates for System Explorer.vi"("CD Name"=w235, "error in (no error)"=w237, "CD Template"=w234, "System Explorer folder"=w233) -> ("error out"=w236:errorcluster)  [unwired: 7 in]
          }
          frame Error {
            n108 = call "System Explorer - Copy Templates for System Explorer.vi"("CD Name"=w239, "error in (no error)"=w242, "CD Template"=w238, "System Explorer folder"=w241) -> ("error out"=w240:errorcluster)  [unwired: 7 in]
          }
        }
      }
      frame "PC-System Explorer - Create extra pages" {
        # "Create a VI for each extra page on the file system."
        n109 = property class="Consolidated_CD"(reference=w246) -> ("Accessors:CD Template"=w245:refnum<class "NIVS_CD Template.lvclass">, "Project Root"=w243:path)  [unwired: 1 in, 2 out]
        n110 = property class="CD Template"(reference=w245) -> ("Accessors:Extra Page Names"=w244:string[])  [unwired: 1 in, 2 out]
        n111 = call-poly "Constants Main.vi"("Action"=CD_System_Explorer_lvlib."LibraryFolderName") -> ("Output"=w254:string)  [unwired: 10 in]
        n112 = call-poly "Constants Main.vi"("Action"=Common."PathToTemplates") -> ("Output"=w250:string)  [unwired: 10 in]
        n113 = String To Path(string=w250) -> (path=w249:path)
        n114 = Build Path(base path=w249, name or relative path=path "Extra Page.vi") -> (appended path=w255:path)
        n115 = Build Path(base path=w243, name or relative path=w254) -> (appended path=w252:path)
        n116 = for "Iterate over all extra pages" {
          tunnel: w244 -> [w259] mode=indexing
          shift-right: [w262] -> w257
          shift-left: w247 -> [w268]
          tunnel: w252 -> [w266]
          tunnel: w255 -> [w267]
          n117 = Concatenate Strings(w259, ".vi") -> (w269:string)
          n118 = Build Path(base path=w266, name or relative path=w269) -> (appended path=w264:path)
          n119 = call "Copy VI and disconnect it from library.vi"("error in (no error)"=w268, "VI Target Path"=w264, "VI Source Path"=w267) -> ("error out"=w265:errorcluster)  [unwired: 8 in]
          n120 = Concatenate Strings(w259, ".htm" ("string")) -> (w261:string)
          n121 = call "Set BD string constant value.vi"("error in (no error)"=w265, "Name of string constant"="CD_CHM_Section", "New String Value"=w261, "Path to VI"=w264) -> ("error out"=w262:errorcluster)  [unwired: 7 in]
        }
      }
      frame "PC-System Explorer - Create library" {
        # "Create the library for System Explorer components."
        n122 = property class="Consolidated_CD"(reference=w273) -> ("Project Name"=w272:string, "Project Root"=w271:path)  [unwired: 1 in, 2 out]
        n123 = call-poly "Constants Main.vi"("Action"=CD_System_Explorer_lvlib."LibraryFolderName") -> ("Output"=w284:string)  [unwired: 10 in]
        n124 = call-poly "Constants Main.vi"("Action"=CD_System_Explorer_lvlib."LibraryFileName") -> ("Output"=w285:string)  [unwired: 10 in]
        n125 = Format Into String(format string=w285, w272) -> (resulting string=w286:string)  [unwired: 2 in, 1 out]
        n126 = Build Path(base path=w271, name or relative path=w284) -> (appended path=w287:path)
        n127 = Build Path(base path=w287, name or relative path=w286) -> (appended path=w276:path)
        n128 = invoke class="App" method="Library.Create"(error in=w274) -> (error out=w279:errorcluster, "Create Library"=w278:refnum<vi>)  [unwired: 3 in, 2 out]
        n129 = invoke class="Library" method="Save"(reference=w278, error in=w279, "Path"=w276) -> (reference out=w277:refnum<vi>, error out=w275:errorcluster)  [unwired: 1 in, 2 out]
        n130 = Bundle By Name(cluster=w280, "System Explorer Library"=w277) -> (w281:T1)
      }
      frame "PC-System Explorer - Add folders and VIs to library" {
        # "Add virtual folders and all VIs to <CD> System Explorer.lvlib"
        n131 = property class="Consolidated_CD"(reference=w296) -> ("Project Root"=w295:path, "Accessors:CD Template"=w292:refnum<class "NIVS_CD Template.lvclass">)  [unwired: 1 in, 2 out]
        n132 = property class="CD Template"(reference=w292) -> ("Accessors:Extra Page Names"=w294:string[], "Accessors:Support Runtime Configuration"=w289:bool)  [unwired: 1 in, 2 out]
        n133 = To More Specific Class(target class=refnum<class "NIVS_PPLCD Template.lvclass"> refnum ("NIVS_PPLCD Template.lvclass"), reference=w292) -> (error out=w291:errorcluster)  [unwired: 1 in, 1 out]
        n134 = case shown="No Error" w291 {
          tunnel: w298 -> [w308 w319]
          tunnel: w297 -> [w305 w317]
          tunnel: [w301 w314] -> w290
          tunnel: w295 -> [w306 w313]
          tunnel: w294 -> [w307 w312]
          tunnel: w289 -> [w300 w309]
          frame No Error {
            n135 = call "System Explorer - Add PPL content to System Explorer library.vi"("Support Runtime Configuration"=w300, "error in (no error)"=w308, "Extra Page Names"=w307, "Project Root"=w306, "CD Wizard - Internal Data"=w305) -> ("error out"=w302:errorcluster, "VIs to Process"=w304:path[], "subVIs to replace"=w303:path[])  [unwired: 4 in]
            n136 = call "Replace Stub SubVIs.vi"("error in"=w302, "VIs to Process"=w304, "subVIs to replace"=w303) -> ("error out"=w301:errorcluster)  [unwired: 8 in]
          }
          frame Error {
            n137 = call "System Explorer - Add content to System Explorer library.vi"("Support Runtime Configuration"=w309, "error in (no error)"=w319, "Extra Page Names"=w312, "Project Root"=w313, "CD Wizard - Internal Data"=w317) -> ("error out"=w318:errorcluster, "Extra Page VIs"=w310:path[], "System Explorer Main VI"=w316:path, "Load Help File VI"=w315:path)  [unwired: 3 in]
            n138 = Build Array (concatenate)(w316, w310) -> (w311:path[])
            n139 = for {
              tunnel: w311 -> [w325] mode=indexing
              tunnel: w315 -> [w324]
              shift-right: [w321] -> w314
              shift-left: w318 -> [w334]
              # "On the diagram of the Main VI and all the Extra Page VIs, replace the stub subVI for Load Help File.vi with the actual new VI."
              n140 = Open VI Reference(vi path=w325, error in (no error)=w334) -> (vi reference=w331:refnum<vi>, error out=w333:errorcluster)  [unwired: 4 in]
              n141 = call <vilib>:"TRef Find Object By Label.vi"("Label"="Load Help File_stub.vi", "Traverse Target"=TRef_TravTarget."BD", "error in (no error)"=w333, "Class Name"="SubVI", "VI Ref"=w331) -> ("error out"=w332:errorcluster, "Found Obj Ref"=w326:refnum<vi>, "dup VI Ref"=w322:refnum<vi>)  [unwired: 3 in, 1 out]
              n142 = invoke class="GObj" method="Replace"(reference=w326, error in=w332, "Path"=w324) -> (error out=w327:errorcluster)  [unwired: 3 in, 5 out]
              n143 = invoke class="VI" method="Save.Instrument"(reference=w322, error in=w327) -> (reference out=w320:refnum<vi>, error out=w323:errorcluster)  [unwired: 4 in, 4 out]
              n144 = Close Reference(reference=w320, error in (no error)=w323) -> (error out=w321:errorcluster)
            }
          }
        }
      }
      frame "PC-Engine - Create folder and copy the RT Template" {
        # "Create a new Engine folder on the file system and copy the RT Driver VI for the chosen custom device."
        n145 = property class="Consolidated_CD"(reference=w339) -> ("Accessors:CD Template"=w336:refnum<class "NIVS_CD Template.lvclass">, "Project Name"=w338:string, "Project Root"=w337:path)  [unwired: 1 in, 2 out]
        n146 = call-dynamic "Create Engine Folder and Copy RT Template.vi"("error in (no error)"=w341, "Project Root"=w337, "Project Name"=w338, "CD Template"=w336) -> ("error out"=w335:errorcluster)  [unwired: 7 in]
      }
      frame "PC-Engine - Create library" {
        # "Create the library for the Engine components."
        n147 = property class="Consolidated_CD"(reference=w345) -> ("Project Name"=w344:string, "Project Root"=w343:path)  [unwired: 1 in, 2 out]
        n148 = call-poly "Constants Main.vi"("Action"=CD_Engine_lvlib."LibraryFolderName") -> ("Output"=w356:string)  [unwired: 10 in]
        n149 = call-poly "Constants Main.vi"("Action"=CD_Engine_lvlib."LibraryFileName") -> ("Output"=w357:string)  [unwired: 10 in]
        n150 = Format Into String(format string=w357, w344) -> (resulting string=w358:string)  [unwired: 2 in, 1 out]
        n151 = Build Path(base path=w343, name or relative path=w356) -> (appended path=w359:path)
        n152 = Build Path(base path=w359, name or relative path=w358) -> (appended path=w347:path)
        n153 = invoke class="App" method="Library.Create"(error in=w346) -> (error out=w351:errorcluster, "Create Library"=w350:refnum<vi>)  [unwired: 3 in, 2 out]
        n154 = invoke class="Library" method="Save"(reference=w350, error in=w351, "Path"=w347) -> (reference out=w348:refnum<vi>, error out=w349:errorcluster)  [unwired: 1 in, 2 out]
        n155 = Bundle By Name(cluster=w353, "Engine Library"=w348) -> (w352:T1)
      }
      frame "PC-Engine - Add virtual folders and VIs to library" {
        # "Add all virtual folders and template VIs to the Engine library"
        n156 = property class="Consolidated_CD"(reference=w366) -> ("Accessors:CD Template"=w364:refnum<class "NIVS_CD Template.lvclass">, "Project Root"=w363:path, "Project Name"=w362:string)  [unwired: 1 in, 2 out]
        n157 = call-dynamic "Add content to Engine library.vi"("Project Name"=w362, "error in (no error)"=w367, "Project Root"=w363, "CD Wizard - Internal Data"=w365, "CD Template"=w364) -> ("error out"=w361:errorcluster)  [unwired: 6 in]
      }
      frame "PC-XML - Create and change file" {
        # "Create the XML file and add it to the project tree"
        n158 = call "XML - Create XML file.vi"("error in (no error)"=w372, "Consolidated_CD"=w370, "CD Wizard - Internal Data"=w371) -> ("error out"=w369:errorcluster)  [unwired: 8 in]
      }
      frame "PC-Help - Copy HTML Files" {
        # "Note: We only copy the files here, the get added to the project in the \"Write New Project File\" case since the project doesn't exist (to add the folder to) until that case."
        # "Copy all of the HTML template files to the new help directory, and configure Build CHM file."
        n159 = property class="Consolidated_CD" props=["Project Name", "Project Root", "Accessors:CD Template"](reference=w377) -> ("Project Root"=w376:path, "Accessors:CD Template"=w375:refnum<class "NIVS_CD Template.lvclass">)  [unwired: 1 in, 3 out]
        n160 = property class="CD Template"(reference=w375) -> ("Accessors:Extra Page Names"=w374:string[])  [unwired: 1 in, 2 out]
        n161 = Build Path(base path=w376, name or relative path=path "Help") -> (appended path=w385:path)
        n162 = call <vilib>:"Check if File or Folder Exists.vi"("error in (no error)"=w387, "path"=w385) -> ("error out"=w388:errorcluster, "file or folder exists?"=w390:bool, "dup path"=w391:path)  [unwired: 7 in]
        n163 = case shown="True" w390 {
          tunnel: w391 -> [w394 w398]
          tunnel: [w394 w397] -> w380
          tunnel: [w393 w396] -> w389
          tunnel: w388 -> [w393 w395]
          frame False {
          }
          frame True {
            n164 = Delete(path (use dialog)=w398, entire hierarchy (F)=TRUE, error in=w395) -> (deleted path=w397:path, error out=w396:errorcluster)  [unwired: 2 in, 1 out]
          }
        }
        n165 = Build Array (concatenate)("Main", w374) -> (w379:string[])
        n166 = Create Folder(path (use dialog)=w380, error in=w389) -> (created path=w382:path, error out=w381:errorcluster)  [unwired: 1 in, 1 out]
        n167 = call "Call HTML Help Generation Functions Async.vi"("error in (no error)"=w381, "Extra Page Names"=w379, "Destination Base Path"=w382) -> ("error out"=w378:errorcluster)  [unwired: 7 in, 1 out]
      }
      frame "Project - Read project file content" {
        w415 = -1  # Read all lines
        w414 = T12."open"  # operation
        w413 = enum16{"read/write", "read-only", "write-only"}."read-only"  # access
        # "Open the project file and read the complete content."
        n168 = property class="Consolidated_CD"(reference=w405) -> ("Accessors:CD Template"=w403:refnum<class "NIVS_CD Template.lvclass">)  [unwired: 1 in, 2 out]
        n169 = To More Specific Class(target class=refnum<class "NIVS_PPLCD Template.lvclass"> refnum ("NIVS_PPLCD Template.lvclass"), reference=w403) -> (error out=w402:errorcluster)  [unwired: 1 in, 1 out]
        n170 = case shown="No Error" w402 {
          tunnel: [w418 w419] -> w408
          frame No Error {
            n171 = call-poly "Constants Main.vi"("Action"=Common."ProjectPPLTemplatePathAndName") -> ("Output"=w418:string)  [unwired: 10 in]
          }
          frame Error {
            n172 = call-poly "Constants Main.vi"("Action"=Common."ProjectTemplatePathAndName") -> ("Output"=w419:string)  [unwired: 10 in]
          }
        }
        n173 = String To Path(string=w408) -> (path=w409:path)
        n174 = Open/Create/Replace File(file path (use dialog)=w409, error in=w406, operation (0:open)=w414, access (0:read/write)=w413) -> (refnum out=w411:refnum<file>, error out=w412:errorcluster)  [unwired: 3 out]
        n175 = Read from Text File(file (use dialog)=w411, count=w415, error in=w412) -> (refnum out=w407:refnum<file>, text=w410:string[], error out=w401:errorcluster)  [unwired: 2 out]
        n176 = Close File(refnum=w407, error in=w401) -> (error out=w400:errorcluster)  [unwired: 1 out]
      }
      frame "Project - Edit Utility section" {
        # "Edit the entries for the utility folder. Also added CHM pre build action entries"
        n177 = property class="Consolidated_CD"(reference=w425) -> ("Accessors:CD Template"=w423:refnum<class "NIVS_CD Template.lvclass">)  [unwired: 1 in, 2 out]
        n178 = To More Specific Class(target class=refnum<class "NIVS_PPLCD Template.lvclass"> refnum ("NIVS_PPLCD Template.lvclass"), reference=w423) -> (error out=w426:errorcluster)  [unwired: 1 in, 1 out]
        n179 = case shown="Error .." w426 {
          tunnel: w424 -> [w440 w469]
          tunnel: [w438 w468] -> w422
          tunnel: [w439 w467] -> w421
          tunnel: w428 -> [w441 w462]
          frame No Error {
            n180 = call-poly "Constants Main.vi"("Action"=Utility_folder."Utility.FolderName") -> ("Output"=w436:string)  [unwired: 10 in]
            n181 = call-poly "Constants Main.vi"("Action"=Utility_folder."Utility.XMLUpdater.FileName") -> ("Output"=w434:string)  [unwired: 10 in]
            n182 = call-poly "Constants Main.vi"("Action"=Utility_folder."Utility.XMLUpdater.FolderName") -> ("Output"=w432:string)  [unwired: 10 in]
            n183 = call-poly "Constants Main.vi"("Action"=Utility_folder."Utility.XMLUpdater.Library.FileName") -> ("Output"=w430:string)  [unwired: 10 in]
            n184 = for "For Iterate over each line and change the placeholders for the Utility entries." {
              tunnel: w440 -> [w456] mode=indexing
              shift-right: [w447] -> w439
              shift-left: w441 -> [w454]
              tunnel: [w446] -> w438 mode=indexing
              tunnel: w434 -> [w455]
              tunnel: w436 -> [w453]
              tunnel: w432 -> [w450]
              tunnel: w430 -> [w445]
              w442 = TRUE  # ignore case?
              w443 = TRUE  # replace all?
              w459 = "%PPLXMLUpdaterFileName%"  # search
              w461 = "%UtilityFolderName%"  # search
              # "Copy .LLB to NI VeriStand dir.vi"
              # "Utility"
              n185 = Search and Replace String(replace all?=w443, case sensitive?=w442, input string=w456, search string=w461, replace string=w453, error in=w454) -> (result string=w460:string, error out=w458:errorcluster)  [unwired: 2 in, 2 out]
              n186 = Search and Replace String(replace all?=w443, case sensitive?=w442, input string=w460, search string=w459, replace string=w455, error in=w458) -> (result string=w452:string, error out=w457:errorcluster)  [unwired: 2 in, 2 out]
              n187 = Search and Replace String(replace all?=w443, case sensitive?=w442, input string=w452, search string="%XMLUpdaterFolderName%" ("result string"), replace string=w450, error in=w457) -> (result string=w449:string, error out=w448:errorcluster)  [unwired: 2 in, 2 out]
              n188 = Search and Replace String(replace all?=w443, case sensitive?=w442, input string=w449, search string="%XMLUpdaterLibraryFileName%" ("result string"), replace string=w445, error in=w448) -> (result string=w446:string, error out=w447:errorcluster)  [unwired: 2 in, 2 out]
            }
          }
          frame Error {
            n189 = call-poly "Constants Main.vi"("Action"=Utility_folder."Utility.FolderName") -> ("Output"=w463:string)  [unwired: 10 in]
            n190 = call-poly "Constants Main.vi"("Action"=Utility_folder."Utility.Copy .llb to NI VeriStand dir.FileName") -> ("Output"=w464:string)  [unwired: 10 in]
            n191 = for "For Iterate over each line and change the placeholders for the Utility entries." {
              tunnel: w469 -> [w476] mode=indexing
              shift-right: [w477] -> w467
              shift-left: w462 -> [w474]
              tunnel: [w472] -> w468 mode=indexing
              tunnel: w464 -> [w475]
              tunnel: w463 -> [w473]
              w470 = TRUE  # ignore case?
              w471 = TRUE  # replace all?
              w479 = "%CopyLLBtoNIVSFileName%"  # search
              w481 = "%UtilityFolderName%"  # search
              # "Copy .LLB to NI VeriStand dir.vi"
              # "Utility"
              n192 = Search and Replace String(replace all?=w471, case sensitive?=w470, input string=w476, search string=w481, replace string=w473, error in=w474) -> (result string=w480:string, error out=w478:errorcluster)  [unwired: 2 in, 2 out]
              n193 = Search and Replace String(replace all?=w471, case sensitive?=w470, input string=w480, search string=w479, replace string=w475, error in=w478) -> (result string=w472:string, error out=w477:errorcluster)  [unwired: 2 in, 2 out]
            }
          }
        }
      }
      frame "Project - Edit XML section" {
        # "Edit the Name and Path for the XML file."
        n194 = property class="Consolidated_CD"(reference=w484) -> ("Project Name"=w483:string, "Accessors:CD Template"=w482:refnum<class "NIVS_CD Template.lvclass">)  [unwired: 1 in, 2 out]
        n195 = call "XML - Get XML file name.vi"("CD Template"=w482, "CD Name"=w483) -> ("XML file name"=w486:string)  [unwired: 9 in]
        n196 = for "Iterate over each line and change the placeholder for the XML file name." {
          tunnel: w489 -> [w497] mode=indexing
          shift-right: [w496] -> w490
          shift-left: w485 -> [w492]
          tunnel: [w495] -> w488 mode=indexing
          tunnel: w486 -> [w491]
          w493 = TRUE  # ignore case?
          w494 = TRUE  # replace all?
          w498 = "%XMLCustomDeviceFileName%"  # search
          n197 = Search and Replace String(replace all?=w494, case sensitive?=w493, input string=w497, search string=w498, replace string=w491, error in=w492) -> (result string=w495:string, error out=w496:errorcluster)  [unwired: 2 in, 2 out]
        }
      }
      frame "Project - Edit Engine Library section" {
        # "Edit the entries for the Engine Library (Library name and folder name)"
        n198 = property class="Consolidated_CD"(reference=w500) -> ("Project Name"=w499:string)  [unwired: 1 in, 2 out]
        n199 = call "Change Engine Library Placeholders in project.vi"("error in (no error)"=w504, "Project Name"=w499, "Project file content in"=w501) -> ("error out"=w503:errorcluster, "Project file content out"=w505:string[])  [unwired: 7 in]
      }
      frame "Project - Edit Shared Library section" {
        # "Edit the entries for the Shared Library (Library name and folder name)"
        n200 = property class="Consolidated_CD"(reference=w507) -> ("Project Name"=w506:string)  [unwired: 1 in, 2 out]
        n201 = call-poly "Constants Main.vi"("Action"=CD_Shared_lvlib."LibraryFileName") -> ("Output"=w515:string)  [unwired: 10 in]
        n202 = call-poly "Constants Main.vi"("Action"=CD_Shared_lvlib."LibraryFolderName") -> ("Output"=w511:string)  [unwired: 10 in]
        n203 = call-poly "Constants Main.vi"("Action"=CD_Shared_lvlib."Shared.FolderName") -> ("Output"=w510:string)  [unwired: 10 in]
        n204 = Format Into String(format string=w515, w506) -> (resulting string=w512:string)  [unwired: 2 in, 1 out]
        n205 = for "Iterate over each line and change the placeholder for the Shared Library file and folder name." {
          tunnel: w513 -> [w534] mode=indexing
          shift-right: [w527] -> w518
          shift-left: w508 -> [w533]
          tunnel: [w528] -> w519 mode=indexing
          tunnel: w512 -> [w522]
          tunnel: w511 -> [w521]
          tunnel: w510 -> [w520]
          w525 = "%SharedLibrarySubfolderName%"  # search
          w531 = "%SharedLibraryFolderName%"  # search
          w523 = TRUE  # ignore case?
          w524 = TRUE  # replace all?
          w535 = "%SharedLibraryFileName%"  # search
          # "Shared"
          # "Shared"
          # "<CD> Shared.lvlib"
          n206 = Search and Replace String(replace all?=w524, case sensitive?=w523, input string=w534, search string=w535, replace string=w522, error in=w533) -> (result string=w532:string, error out=w530:errorcluster)  [unwired: 2 in, 2 out]
          n207 = Search and Replace String(replace all?=w524, case sensitive?=w523, input string=w532, search string=w531, replace string=w521, error in=w530) -> (result string=w529:string, error out=w526:errorcluster)  [unwired: 2 in, 2 out]
          n208 = Search and Replace String(replace all?=w524, case sensitive?=w523, input string=w529, search string=w525, replace string=w520, error in=w526) -> (result string=w528:string, error out=w527:errorcluster)  [unwired: 2 in, 2 out]
        }
      }
      frame "Project - Edit System Explorer Library section" {
        # "Edit the entries for the System Explorer Library (Library name and folder name)"
        n209 = property class="Consolidated_CD"(reference=w538) -> ("Project Name"=w537:string)  [unwired: 1 in, 2 out]
        n210 = call-poly "Constants Main.vi"("Action"=CD_System_Explorer_lvlib."LibraryFileName") -> ("Output"=w544:string)  [unwired: 10 in]
        n211 = Format Into String(format string=w544, w537) -> (resulting string=w547:string)  [unwired: 2 in, 1 out]
        n212 = call-poly "Constants Main.vi"("Action"=CD_System_Explorer_lvlib."System Explorer.FolderName") -> ("Output"=w549:string)  [unwired: 10 in]
        n213 = call-poly "Constants Main.vi"("Action"=CD_System_Explorer_lvlib."LibraryFolderName") -> ("Output"=w548:string)  [unwired: 10 in]
        n214 = for "Iterate over each line and change the placeholder for the System Explorer Library file and folder name." {
          tunnel: w541 -> [w564] mode=indexing
          shift-right: [w556] -> w542
          shift-left: w539 -> [w563]
          tunnel: [w557] -> w536 mode=indexing
          tunnel: w547 -> [w552]
          tunnel: w548 -> [w551]
          tunnel: w549 -> [w550]
          w553 = "%SystemExplorerSubfolderName%"  # search
          w561 = "%SystemExplorerLibraryFolderName%"  # search
          w555 = TRUE  # ignore case?
          w554 = TRUE  # replace all?
          w565 = "%SystemExplorerLibraryFileName%"  # search
          n215 = Search and Replace String(replace all?=w554, case sensitive?=w555, input string=w564, search string=w565, replace string=w552, error in=w563) -> (result string=w562:string, error out=w560:errorcluster)  [unwired: 2 in, 2 out]
          n216 = Search and Replace String(replace all?=w554, case sensitive?=w555, input string=w562, search string=w561, replace string=w551, error in=w560) -> (result string=w558:string, error out=w559:errorcluster)  [unwired: 2 in, 2 out]
          n217 = Search and Replace String(replace all?=w554, case sensitive?=w555, input string=w558, search string=w553, replace string=w550, error in=w559) -> (result string=w557:string, error out=w556:errorcluster)  [unwired: 2 in, 2 out]
        }
      }
      frame "Project - Edit Custom Device Name" {
        # "Edit the Custom Device name"
        n218 = property class="Consolidated_CD"(reference=w567) -> ("Project Name"=w566:string)  [unwired: 1 in, 2 out]
        n219 = for "Iterate over each line and change the placeholder for the Custom Device name." {
          tunnel: w569 -> [w579] mode=indexing
          shift-right: [w574] -> w571
          shift-left: w572 -> [w575]
          tunnel: [w578] -> w570 mode=indexing
          tunnel: w566 -> [w573]
          w576 = TRUE  # ignore case?
          w577 = TRUE  # replace all?
          w580 = "%CustomDeviceName%"  # search
          # "<CD>"
          n220 = Search and Replace String(replace all?=w577, case sensitive?=w576, input string=w579, search string=w580, replace string=w573, error in=w575) -> (result string=w578:string, error out=w574:errorcluster)  [unwired: 2 in, 2 out]
        }
      }
      frame "Project - Edit System Explorer LLB Name" {
        # "Edit the name for the System Explorer LLB."
        n221 = property class="Consolidated_CD"(reference=w583) -> ("Project Name"=w585:string, "Accessors:CD Template"=w581:refnum<class "NIVS_CD Template.lvclass">)  [unwired: 1 in, 2 out]
        n222 = To More Specific Class(target class=refnum<class "NIVS_PPLCD Template.lvclass"> refnum ("NIVS_PPLCD Template.lvclass"), reference=w581) -> (error out=w582:errorcluster)  [unwired: 1 in, 1 out]
        n223 = case shown="No Error" w582 {
          tunnel: [w598 w614] -> w590
          tunnel: w588 -> [w594 w610]
          tunnel: [w593 w609] -> w587
          tunnel: w586 -> [w592 w608]
          tunnel: w585 -> [w591 w607]
          frame No Error {
            n224 = call-poly "Constants Main.vi"("Action"=Build_Spec_System_Explorer."Destinations.PPLFileName") -> ("Output"=w597:string)  [unwired: 10 in]
            n225 = Format Into String(format string=w597, w591) -> (resulting string=w595:string)  [unwired: 2 in, 1 out]
            n226 = for "Iterate over each line and change the placeholder for the System Explorer LLB." {
              tunnel: w595 -> [w604]
              tunnel: w594 -> [w602] mode=indexing
              tunnel: [w601] -> w593 mode=indexing
              shift-right: [w600] -> w598
              shift-left: w592 -> [w603]
              w599 = "%SystemExplorerPPLFileName%"  # search
              w605 = TRUE  # ignore case?
              w606 = TRUE  # replace all?
              # "<CD> Configuration.lvlibp"
              n227 = Search and Replace String(replace all?=w606, case sensitive?=w605, input string=w602, search string=w599, replace string=w604, error in=w603) -> (result string=w601:string, error out=w600:errorcluster)  [unwired: 1 in, 3 out]
            }
          }
          frame Default {
            n228 = call-poly "Constants Main.vi"("Action"=Build_Spec_System_Explorer."Destinations.LLBFileName") -> ("Output"=w613:string)  [unwired: 10 in]
            n229 = Format Into String(format string=w613, w607) -> (resulting string=w611:string)  [unwired: 2 in, 1 out]
            n230 = for "Iterate over each line and change the placeholder for the System Explorer LLB." {
              tunnel: w611 -> [w620]
              tunnel: w610 -> [w618] mode=indexing
              tunnel: [w617] -> w609 mode=indexing
              shift-right: [w616] -> w614
              shift-left: w608 -> [w619]
              w615 = "%SystemExplorerLLBFileName%"  # search
              w621 = TRUE  # ignore case?
              w622 = TRUE  # replace all?
              # "<CD> Configuration.llb"
              n231 = Search and Replace String(replace all?=w622, case sensitive?=w621, input string=w618, search string=w615, replace string=w620, error in=w619) -> (result string=w617:string, error out=w616:errorcluster)  [unwired: 1 in, 3 out]
            }
          }
        }
      }
      frame "Project - Edit Engine LLB OS dependent file name" {
        n232 = property class="Consolidated_CD"(reference=w625) -> ("Project Name"=w628:string, "Accessors:CD Template"=w623:refnum<class "NIVS_CD Template.lvclass">)  [unwired: 1 in, 2 out]
        n233 = To More Specific Class(target class=refnum<class "NIVS_PPLCD Template.lvclass"> refnum ("NIVS_PPLCD Template.lvclass"), reference=w623) -> (error out=w624:errorcluster)  [unwired: 1 in, 1 out]
        n234 = case shown="Default" w624 {
          tunnel: w631 -> [w642 w668]
          tunnel: [w641 w667] -> w630
          tunnel: w629 -> [w636 w662]
          tunnel: w628 -> [w635 w661]
          tunnel: [w634 w660] -> w627
          frame No Error {
            n235 = call-poly "Constants Main.vi"("Action"=Build_Spec_Engine."Destinations.PPLLinux64FileName") -> ("Output"=w640:string)  [unwired: 10 in]
            n236 = call-poly "Constants Main.vi"("Action"=Build_Spec_Engine."Destinations.PPLWindowsFileName") -> ("Output"=w644:string)  [unwired: 10 in]
            n237 = Format Into String(format string=w640, w635) -> (resulting string=w633:string)  [unwired: 2 in, 1 out]
            n238 = Format Into String(format string=w644, w635) -> (resulting string=w638:string)  [unwired: 2 in, 1 out]
            n239 = Build Array(w638, w633) -> (w637:string[])
            n240 = for {
              shift-right: [w649] -> w641
              shift-left: w636 -> [w650]
              tunnel: w642 -> [w646] mode=indexing
              tunnel: w637 -> [w647]
              tunnel: [w645] -> w634 mode=indexing
              n241 = for {
                shift-right: [w658] -> w649
                shift-left: w650 -> [w657]
                shift-right: [w654] -> w645
                shift-left: w646 -> [w653]
                tunnel: string[] ["%EnginePPLWindowsFileName%", "%EnginePPLLinux64FileName%"] -> [w652] mode=indexing
                tunnel: w647 -> [w651] mode=indexing
                w655 = TRUE  # ignore case?
                w656 = TRUE  # replace all?
                n242 = Search and Replace String(replace all?=w656, case sensitive?=w655, input string=w653, search string=w652, replace string=w651, error in=w657) -> (result string=w654:string, error out=w658:errorcluster)  [unwired: 1 in, 3 out]
              }
            }
          }
          frame Default {
            n243 = call-poly "Constants Main.vi"("Action"=Build_Spec_Engine."Destinations.LLBLinux64FileName") -> ("Output"=w666:string)  [unwired: 10 in]
            n244 = call-poly "Constants Main.vi"("Action"=Build_Spec_Engine."Destinations.LLBWindowsFileName") -> ("Output"=w670:string)  [unwired: 10 in]
            n245 = Format Into String(format string=w666, w661) -> (resulting string=w659:string)  [unwired: 2 in, 1 out]
            n246 = Format Into String(format string=w670, w661) -> (resulting string=w664:string)  [unwired: 2 in, 1 out]
            n247 = Build Array(w664, w659) -> (w663:string[])
            n248 = for {
              shift-right: [w675] -> w667
              shift-left: w662 -> [w676]
              tunnel: w668 -> [w672] mode=indexing
              tunnel: w663 -> [w673]
              tunnel: [w671] -> w660 mode=indexing
              n249 = for {
                shift-right: [w684] -> w675
                shift-left: w676 -> [w683]
                shift-right: [w680] -> w671
                shift-left: w672 -> [w679]
                tunnel: string[] ["%EngineLLBWindowsFileName%", "%EngineLLBLinux64FileName%"] -> [w678] mode=indexing
                tunnel: w673 -> [w677] mode=indexing
                w681 = TRUE  # ignore case?
                w682 = TRUE  # replace all?
                n250 = Search and Replace String(replace all?=w682, case sensitive?=w681, input string=w679, search string=w678, replace string=w677, error in=w683) -> (result string=w680:string, error out=w684:errorcluster)  [unwired: 1 in, 3 out]
              }
            }
          }
        }
      }
      frame "Project - Copy Configuration file" {
        n251 = property class="Consolidated_CD"(reference=w692) -> ("Project Name"=w694:string, "Project Root"=w693:path)  [unwired: 1 in, 2 out]
        n252 = call-poly "Constants Main.vi"("Action"=Common."ProjectConfigurationName") -> ("Output"=w695:string)  [unwired: 10 in]
        n253 = Format Into String(format string=w695, w694) -> (resulting string=w697:string)  [unwired: 2 in, 1 out]
        n254 = call-poly "Constants Main.vi"("Action"=Common."PathToConfigurationFile") -> ("Output"=w690:string)  [unwired: 10 in]
        n255 = Build Path(base path=w693, name or relative path=w697) -> (appended path=w688:path)
        n256 = String To Path(string=w690) -> (path=w689:path)
        n257 = Copy(8:w687, 9:FALSE ("overwrite (F)"), 10:w688, 11:w689) -> (0:w686:errorcluster)  [unwired: 1 in, 2 out]
      }
      frame "Project - Write new project file" {
        # "Create new file and write the project file content into it."
        n258 = property class="Consolidated_CD"(reference=w704) -> ("Project Name"=w703:string, "Project Root"=w702:path)  [unwired: 1 in, 2 out]
        n259 = call-poly "Constants Main.vi"("Action"=Common."ProjectName") -> ("Output"=w727:string)  [unwired: 10 in]
        n260 = Format Into String(format string=w727, w703) -> (resulting string=w738:string)  [unwired: 2 in, 1 out]
        n261 = Build Path(base path=w702, name or relative path=w738) -> (appended path=w733:path)
        n262 = Open/Create/Replace File(file path (use dialog)=w733, error in=w705, operation (0:open)=T12."replace or create") -> (refnum out=w735:refnum<file>, error out=w734:errorcluster)  [unwired: 3 in, 1 out]
        n263 = Write to Text File(file (use dialog)=w735, text=w730, error in=w734) -> (refnum out=w732:refnum<file>, error out=w731:errorcluster)  [unwired: 2 out]
        n264 = Close File(refnum=w732, error in=w731) -> (path=w728:path, error out=w726:errorcluster)
        n265 = invoke class="App" method="Project.Open"(error in=w726, "Path"=w728) -> (error out=w721:errorcluster, "Project:Open"=w720:refnum<vi>)  [unwired: 2 in, 2 out]
        n266 = Build Path(base path=w702, name or relative path=path "Help") -> (appended path=w714:path)
        n267 = property class="Project"(reference=w720, error in=w721) -> (reference out=w719:refnum<vi>, error out=w717:errorcluster, "My Computer"=w718:refnum<vi>)
        n268 = invoke class="TargetItem" method="AddItem"(reference=w718, error in=w717, "Name"="Placeholder", "Path"=path "", "Type"="Folder") -> (reference out=w708:refnum<vi>, error out=w724:errorcluster, "AddItem"=w723:refnum<vi>)  [unwired: 1 in, 3 out]
        n269 = invoke class="ProjectItem" method="Convert to Auto-populating Folder"(reference=w723, error in=w724, "Path"=w714) -> (reference out=w710:refnum<vi>, error out=w706:errorcluster)  [unwired: 1 in, 2 out]
        n270 = invoke class="Project" method="Open Window"(reference=w719, error in=w706) -> (reference out=w707:refnum<vi>, error out=w711:errorcluster)  [unwired: 1 in, 1 out]
        n271 = invoke class="Project" method="Save"(reference=w707, error in=w711) -> (reference out=w713:refnum<vi>, error out=w701:errorcluster)  [unwired: 2 in, 2 out]
        n272 = Close Reference(reference=w710, error in (no error)=w701) -> (error out=w709:errorcluster)
        n273 = Close Reference(reference=w708, error in (no error)=w709) -> (error out=w700:errorcluster)
        n274 = Close Reference(reference=w713, error in (no error)=w700) -> (error out=w712:errorcluster)
      }
    }
  }
  "error out" <- w6
